vi "eyecat MAX v02_JS_140204.vi"() -> ()   [LabVIEW 2014]
doc: "This VI is an upgrade from the WIN 1_v4 that implements the ageing subrutine"
uses:
  <vilib>/Utility/file.llb/Write To Spreadsheet File (string).vi
  <vilib>/Utility/file.llb/Read From Spreadsheet File (string).vi
  <vilib>/regexp/Match Regular Expression.xnode
  Controls Win/Control 3.ctl
  <vilib>/Utility/miscctls.llb/LVRowAndColumnTypeDef.ctl
  <vilib>/Platform/TimedLoop/XDataNode/XDataNode.xnode
  <vilib>/Platform/TimedLoop/XDataNode/nitl_modes.ctl
  <vilib>/Platform/TimedLoop/XDataNode/XDNodeRunTimeDep.lvlib
  <vilib>/Platform/TimedLoop/XDataNode/wakeup.ctl
  <vilib>/Platform/TimedLoop/XDataNode/timing_clust.ctl
  Buttons/Numeric control.ctl
  <vilib>/Utility/file.llb/Read From Spreadsheet File (DBL).vi
  Buttons/String input.ctl
  Buttons/Numeric indicator.ctl
  Buttons/String output.ctl
panel:
  in  "MKS":bool
  out "output cluster":T2
  out "Lambda":dbl[](array[numeric])
  out "MKS HC":dbl
  in  "HC Index":i32
  in  "MFC Number":i32
  out "Open/Closed \nLoop":dbl[](array[numeric])
  out "Air Cyc 2":dbl[](array[numeric])
  in  "Cycle size":i32
  out "MFC Setpoint/Delivery":dynamicdata(graph)
  out "ExtAnDn":bool
  out "ExtAnUp":bool
  out "HC Cyc 2":dbl[](array[numeric])
  out "SO Valve 2":dbl[](array[numeric])
  out "SO Valve 1":dbl[](array[numeric])
  out "Air Bal":dbl[](array[numeric])
  out "HC Bal":dbl[](array[numeric])
  out "Air Cyc 1":dbl[](array[numeric])
  out "HC Cyc 1":dbl[](array[numeric])
  out "File name":string
  out "Log?":bool
  out "Advanced Logging":bool
  out "Connected":bool
  out "MKS 1":i16
  out "MKS 2":i16
  out "Furnace temp 2":dbl
  out "Full system?":bool
  out "Log interval (seconds)":T1
  in  "Flow rate Age":dbl
  in  "Inlet temp Age":dbl
  out "Stopped?":bool
  in  "Stop Cmd":T1
  out "Connected?":bool
  out "Error":dbl
  out "Iteration Duration":i64
  out "Finished Late? [i-1]":bool
  in  "stop TCP":bool
  in  "SO2 ppm":dbl
  out "Furnace temp 1":dbl
  out "stop 2":bool
  in  "Enum 1":i16=1
  in  "Acknowledge":bool
  out "Test number":u16
  out "Flag1":bool=TRUE
  out "EditPos Subc":T3
  out "Flag 2":bool=TRUE
  in  "Tab Control":T4(tab)
  out "Doors Unlocked":bool
  in  "Temperature Limit (°C)":T1=800.0 min=0.0 max=1200.0 step=1.0
  in  "Log Test Button":bool
  in  "File Name":T5="Test"
  in  "File Path":path=path "C:/DATA LOG"
  out "Fail":bool
  out "Pass":bool
  in  "Select Test Type":T6(radio)
  out "Standby":bool
  out "Doors Open":bool
  out "Extractor Fan On":bool
  out "Test In Progress":bool
  out "Cool Down":bool
  out "System Alarm":bool
  in  "Execute Leak Test Button":bool
  in  "Stop Test Button":bool
  in  "Start Test Button":bool
  in  "Advanced settings":bool
  in  "Inlet Temperature (°C)":T1=400.0 min=350.0 max=1000.0 step=1.0
  in  "Inlet LAMBDA Rich":T1=0.9 min=0.85 max=0.96 step=0.001
  in  "Inlet LAMBDA Lean":T1=1.2 min=1.02 max=3.0 step=0.001
  in  "Test Stop temperature (°C)":T1=300.0 min=100.0 max=1000.0 step=1.0
  in  "Test Start Temperature (°C)":T1=125.0 min=0.0 max=500.0 step=1.0
  in  "Furnace Ramp Rate (°C/min)":T1=15.0 min=1.0 max=50.0 step=0.1
  in  "NO:CO Ratio":T1=1.1 min=1.0 max=5.0 step=0.1
  in  "Inlet O2 (%)":T1=0.5 min=0.0 max=14.0 step=0.01
  in  "Inlet LAMBDA":T1=1.0 min=0.6 max=3.0 step=0.001
  out "Space Velocity (h-1)":T7
  out "Vol Flow @ STP (l/min)":T7
  in  "Test Flow Rate(g/s)":T1 min=0.0 max=100.0 step=0.01
  out "Sample Volume (litres)":T7
  in  "Number of Samples":T1=1.0 min=1.0 max=6.0 step=1.0
  in  "Sample Diameter (mm)":T1
  out "CO Theory (%)":T7 format="%#_3g"
  out "CO Theory (%)":T7 format="%#_3g"
  out "HC Theory (%)":T7
  in  "Sample Length (mm)":T1 min=0.0 step=0.5
  in  "NO ppm SW":dbl=500.0 caption="NO (ppm)" min=0.0 max=500.0 step=1.0
  in  "NO ppm Loff":T1 caption="NO ppm"
  in  "Delete sCycle":bool
  in  "Load sCycle":bool
  in  "Save sCycle":bool
  in  "Clear subcycle":bool
  in  "Clear Cycle Pattern":bool
  in  "Save Cycle":bool
  in  "Load Cycle":bool
  in  "Delete Cycle":bool
  out "Test Compiled":bool
  in  "Compile Test Button":bool
  in  "Sub-Cycle List":i32(listbox)=1
  in  "Cycle List":i32(listbox)=2
  out "Total Test Duration (hrs)":T8
  in  "Ageing Gas":enum32{"Radio Selection 1", "Radio Selection 2"}(radio)
  in  "Sub-Cycle Pattern":string[][](table) caption="Subcycle pattern"
  in  "Total Number of Cycles":T1=1.0 min=1.0 max=10000.0 step=1.0
  in  "Cycle Pattern":string[][](table)
  in  "Sub-Cycle Name":T5
  in  "Cycle Name":T5
  out "Heat Exchanger Temperatures (°C)":dynamicdata(graph)
  out "Flow Rate (g/s)":dynamicdata(graph)
  out "Sample Temperatures (°C)":dynamicdata(graph)
  out "System Temperatures (°C)":dynamicdata(graph)
  out "HC Concentration (ppm)":dynamicdata(graph)
  out "Lambda":dynamicdata(graph)
  out "M584L Upstream & Downstream":dynamicdata(graph)
  out "NO Concentration (ppm)":dynamicdata(graph)
  in  "Purge System":bool
  in  "Alarm ack":bool
  in  "Clear log":bool
  out "Table":string[][](table)
  out "Soft Alarm":bool
  out "Hard Alarm":bool
  # "0 HC Cyc 1\n1 Air Cyc 1\n2 Air Bal\n3 HC Bal\n4 Air Cyc 2\n5 HC Cyc 2"
  # "Test Type"
  # "Test Commands"
  # "System Indicators"
  # "Leak Test"
  # "Catalyst Specification"
  # "Lightoff Settings"
  # "Furnace Lightoff Settings"
  # "Sweep Settings"
  # "CO/HC Lightoff Settings"
  # "0.96 < lambda < 0.85"
  # "1.02< lambda < 1.6"
  # "350 < Tinlet < 1000"
  # "NO Lightoff Settings"
  # "Flow Specification"
  # "Cycle Compiled"
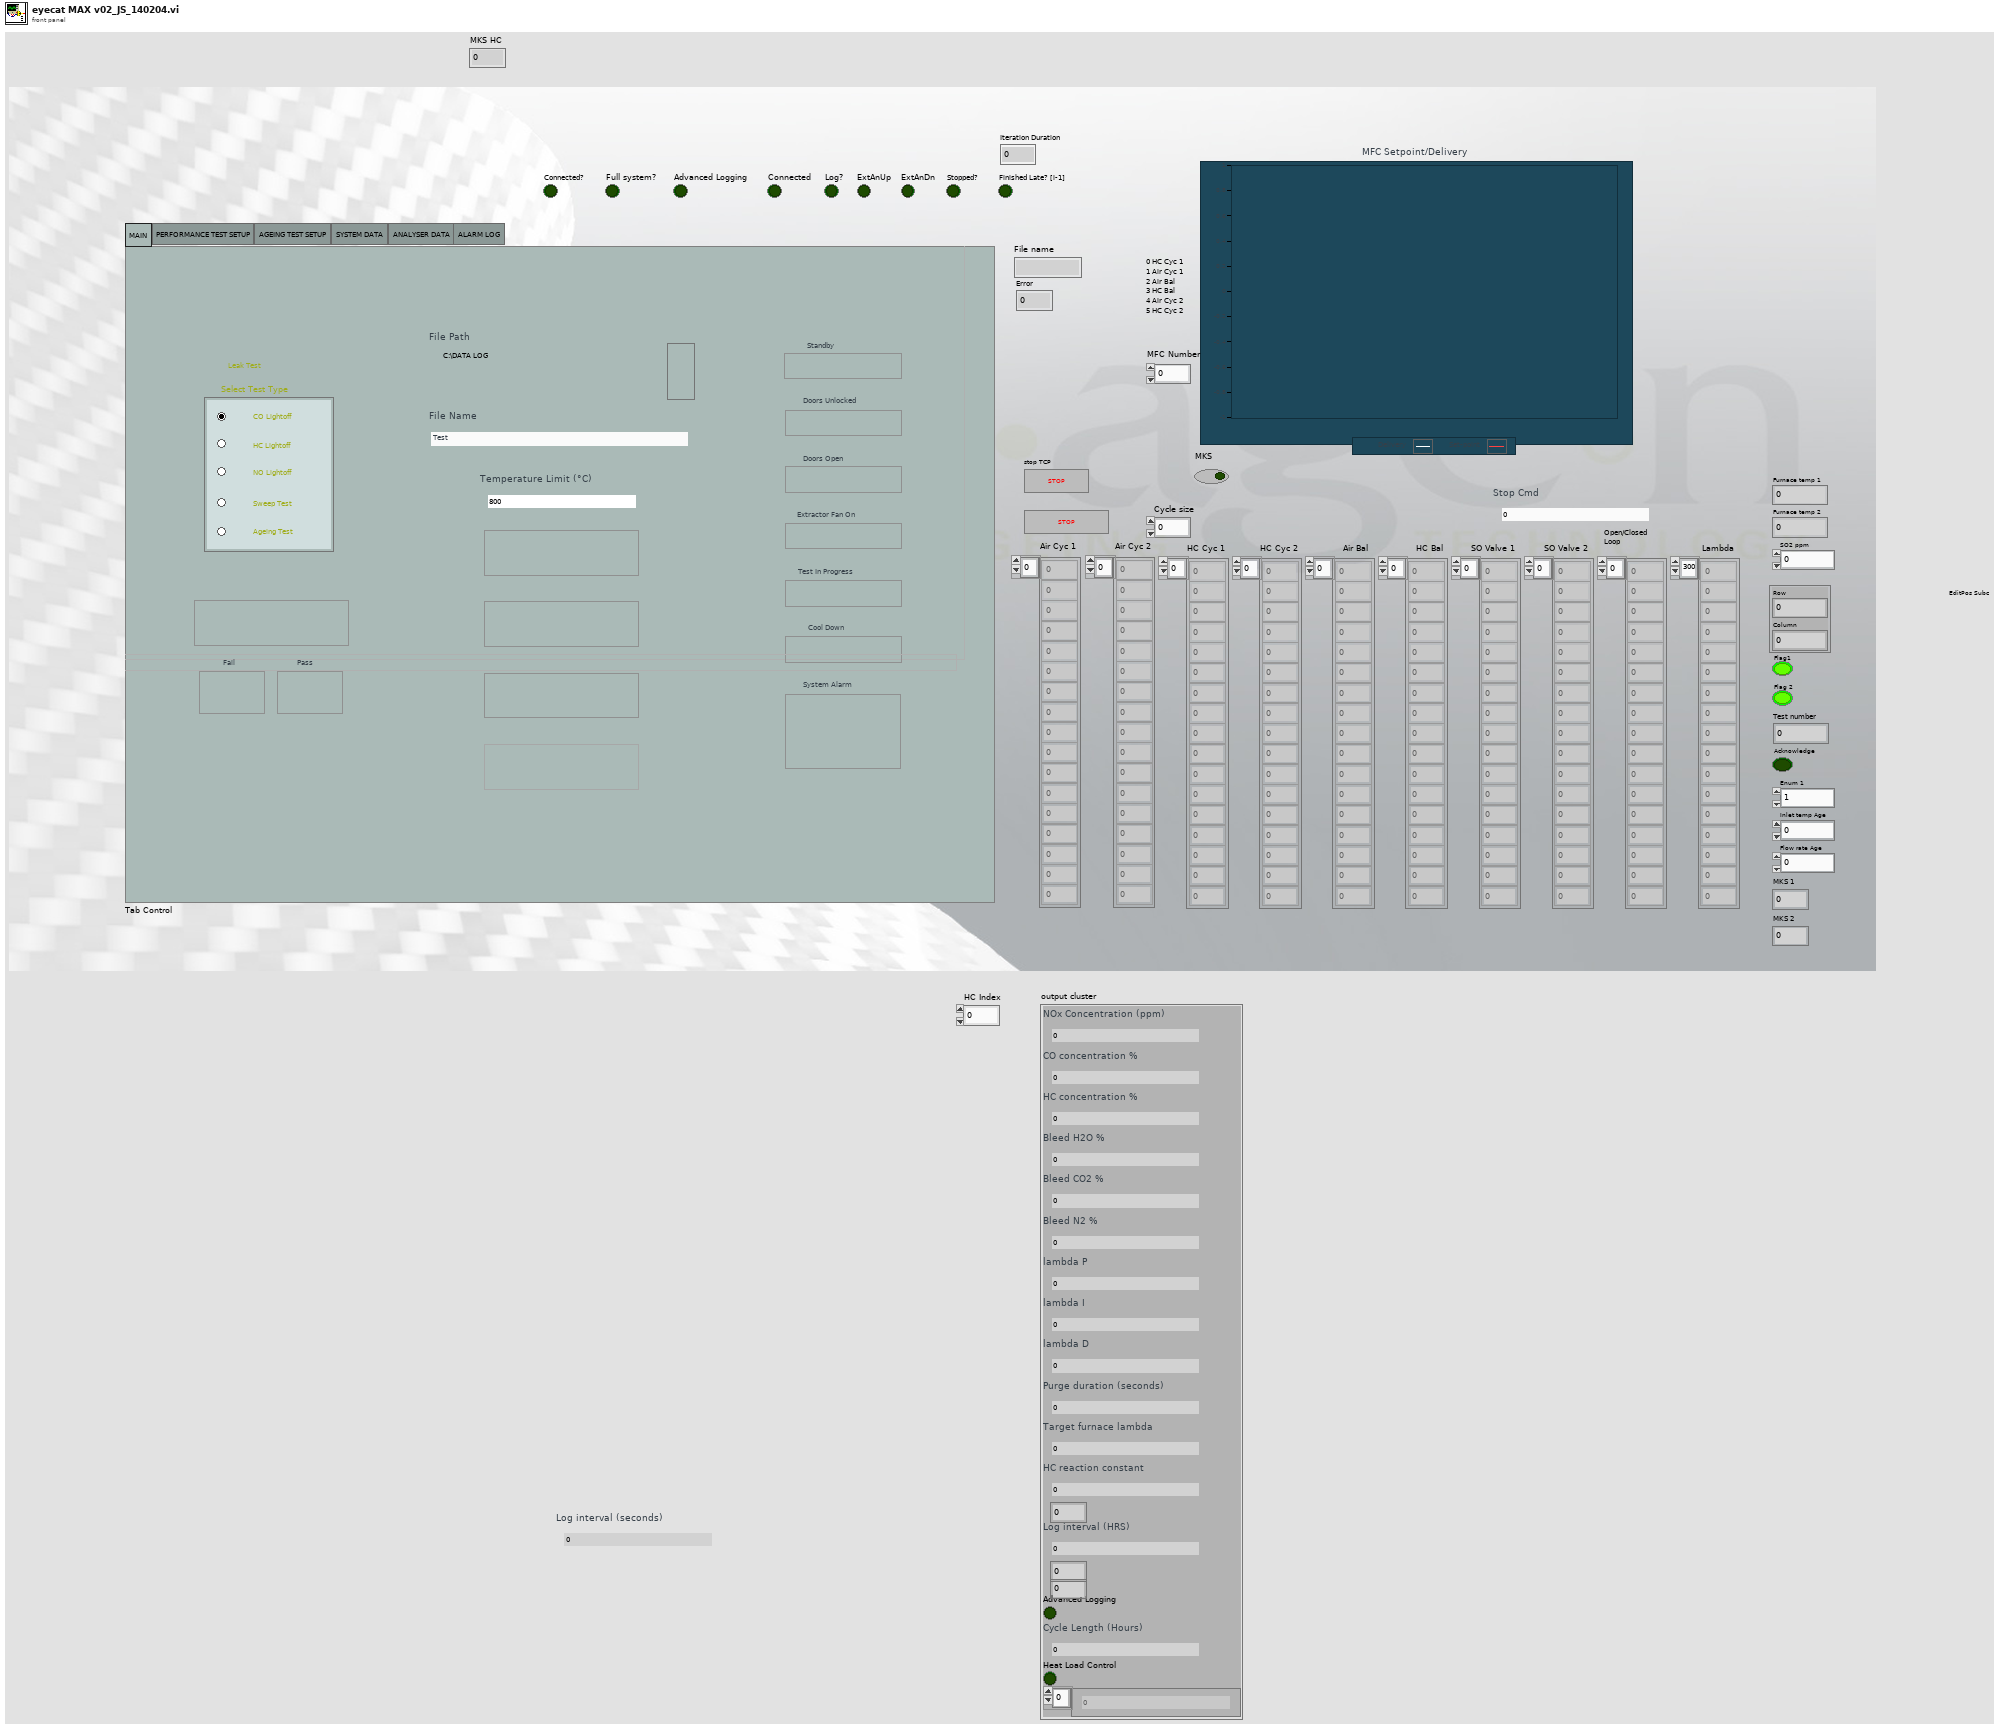
[diagram p1: front panel]
types:
  T1 = typedef "Numeric control.ctl" = dbl
  T2 = cluster{"NOx Concentration (ppm)":T1, "CO concentration %":T1, "HC concentration %":T1, "Bleed H2O %":T1, "Bleed CO2 %":T1, "Bleed N2 %":T1, "lambda P":T1, "lambda I":T1, "lambda D":T1, "Purge duration (seconds)":T1, "Target furnace lambda":T1, "HC reaction constant":T1, i16, "Log interval (HRS)":T1, i16, i16, "Advanced Logging":bool, "Cycle Length (Hours)":T1, "Heat Load Control":bool, T1[]}
  T3 = typedef "LVRowAndColumnTypeDef.ctl" = cluster{"Row":i32, "Column":i32}
  T4 = enum32{"MAIN", "PERFORMANCE TEST SETUP", "AGEING TEST SETUP", "SYSTEM DATA", "ANALYSER DATA", "ALARM LOG"}
  T5 = typedef "String input.ctl" = string
  T6 = enum32{"CO Lightoff", "HC Lightoff", "NO Lightoff", "Sweep Test", "Ageing Test"}
  T7 = typedef "Numeric indicator.ctl" = dbl
  T8 = typedef "String output.ctl" = string
  T9 = typedef "XDNodeRunTimeDep.lvlib/nitl_modes.ctl" = enum32{"No Change", "Process missed periods, maintain original phase", "Discard missed periods, maintain original phase", "Process missed periods, ignore original phase", "Discard missed periods, ignore original phase"}
  T10 = typedef "Control 3.ctl" = enum16{"main", "start test", "save subc", "load subc", "delete subc", "clear table 1", "update list 1", "save cycle", "load cycle", "delete cycle", "clear table 2", "update list 2", "calc HC CO", "Total time calc", "update Cycle pattern ", "load cycle name", "convert to num", "load test array", "check scycle name", "check cycle name", "Multigas connect", "Multigas disconnect"}
  T11 = enum8{"Enabled", "Disabled", "Disabled and Grayed Out"}
  T12 = typedef "XDNodeRunTimeDep.lvlib/timing_clust.ctl" = cluster{"Expected End [f-1]":u64, "Actual End [f-1]":u64, "Finished Late? [f-1]":bool, "Expected End [i-1]":u64, "Actual End [i-1]":u64, "Finished Late? [i-1]":bool, "Expected Start [i]":u64, "Actual Start [i]":u64, "Expected Start [f]":u64, "Actual Start [f]":u64, "Source Name":string, "Structure Name":string, "Period":i64, "Deadline":i64, "Offset":i64, "Start":i64, "Priority":i32, "Timeout":i32, "Mode":T9, "Wakeup Reason":T13, "Error":errorcluster, "Source Type":string, "Secondary Source Type":string, "Global End Time":u64, "Global Start Time":u64, "Frame Duration":u64, "Iteration Duration":u64, "Assigned CPU":i32, "I/O Scan Engine Mode":u32}
  T13 = typedef "XDNodeRunTimeDep.lvlib/wakeup.ctl" = enum32{"Normal", "Aborted", "Asynchronous wakeup", "Timing source error", "Timed loop error", "Timeout"}
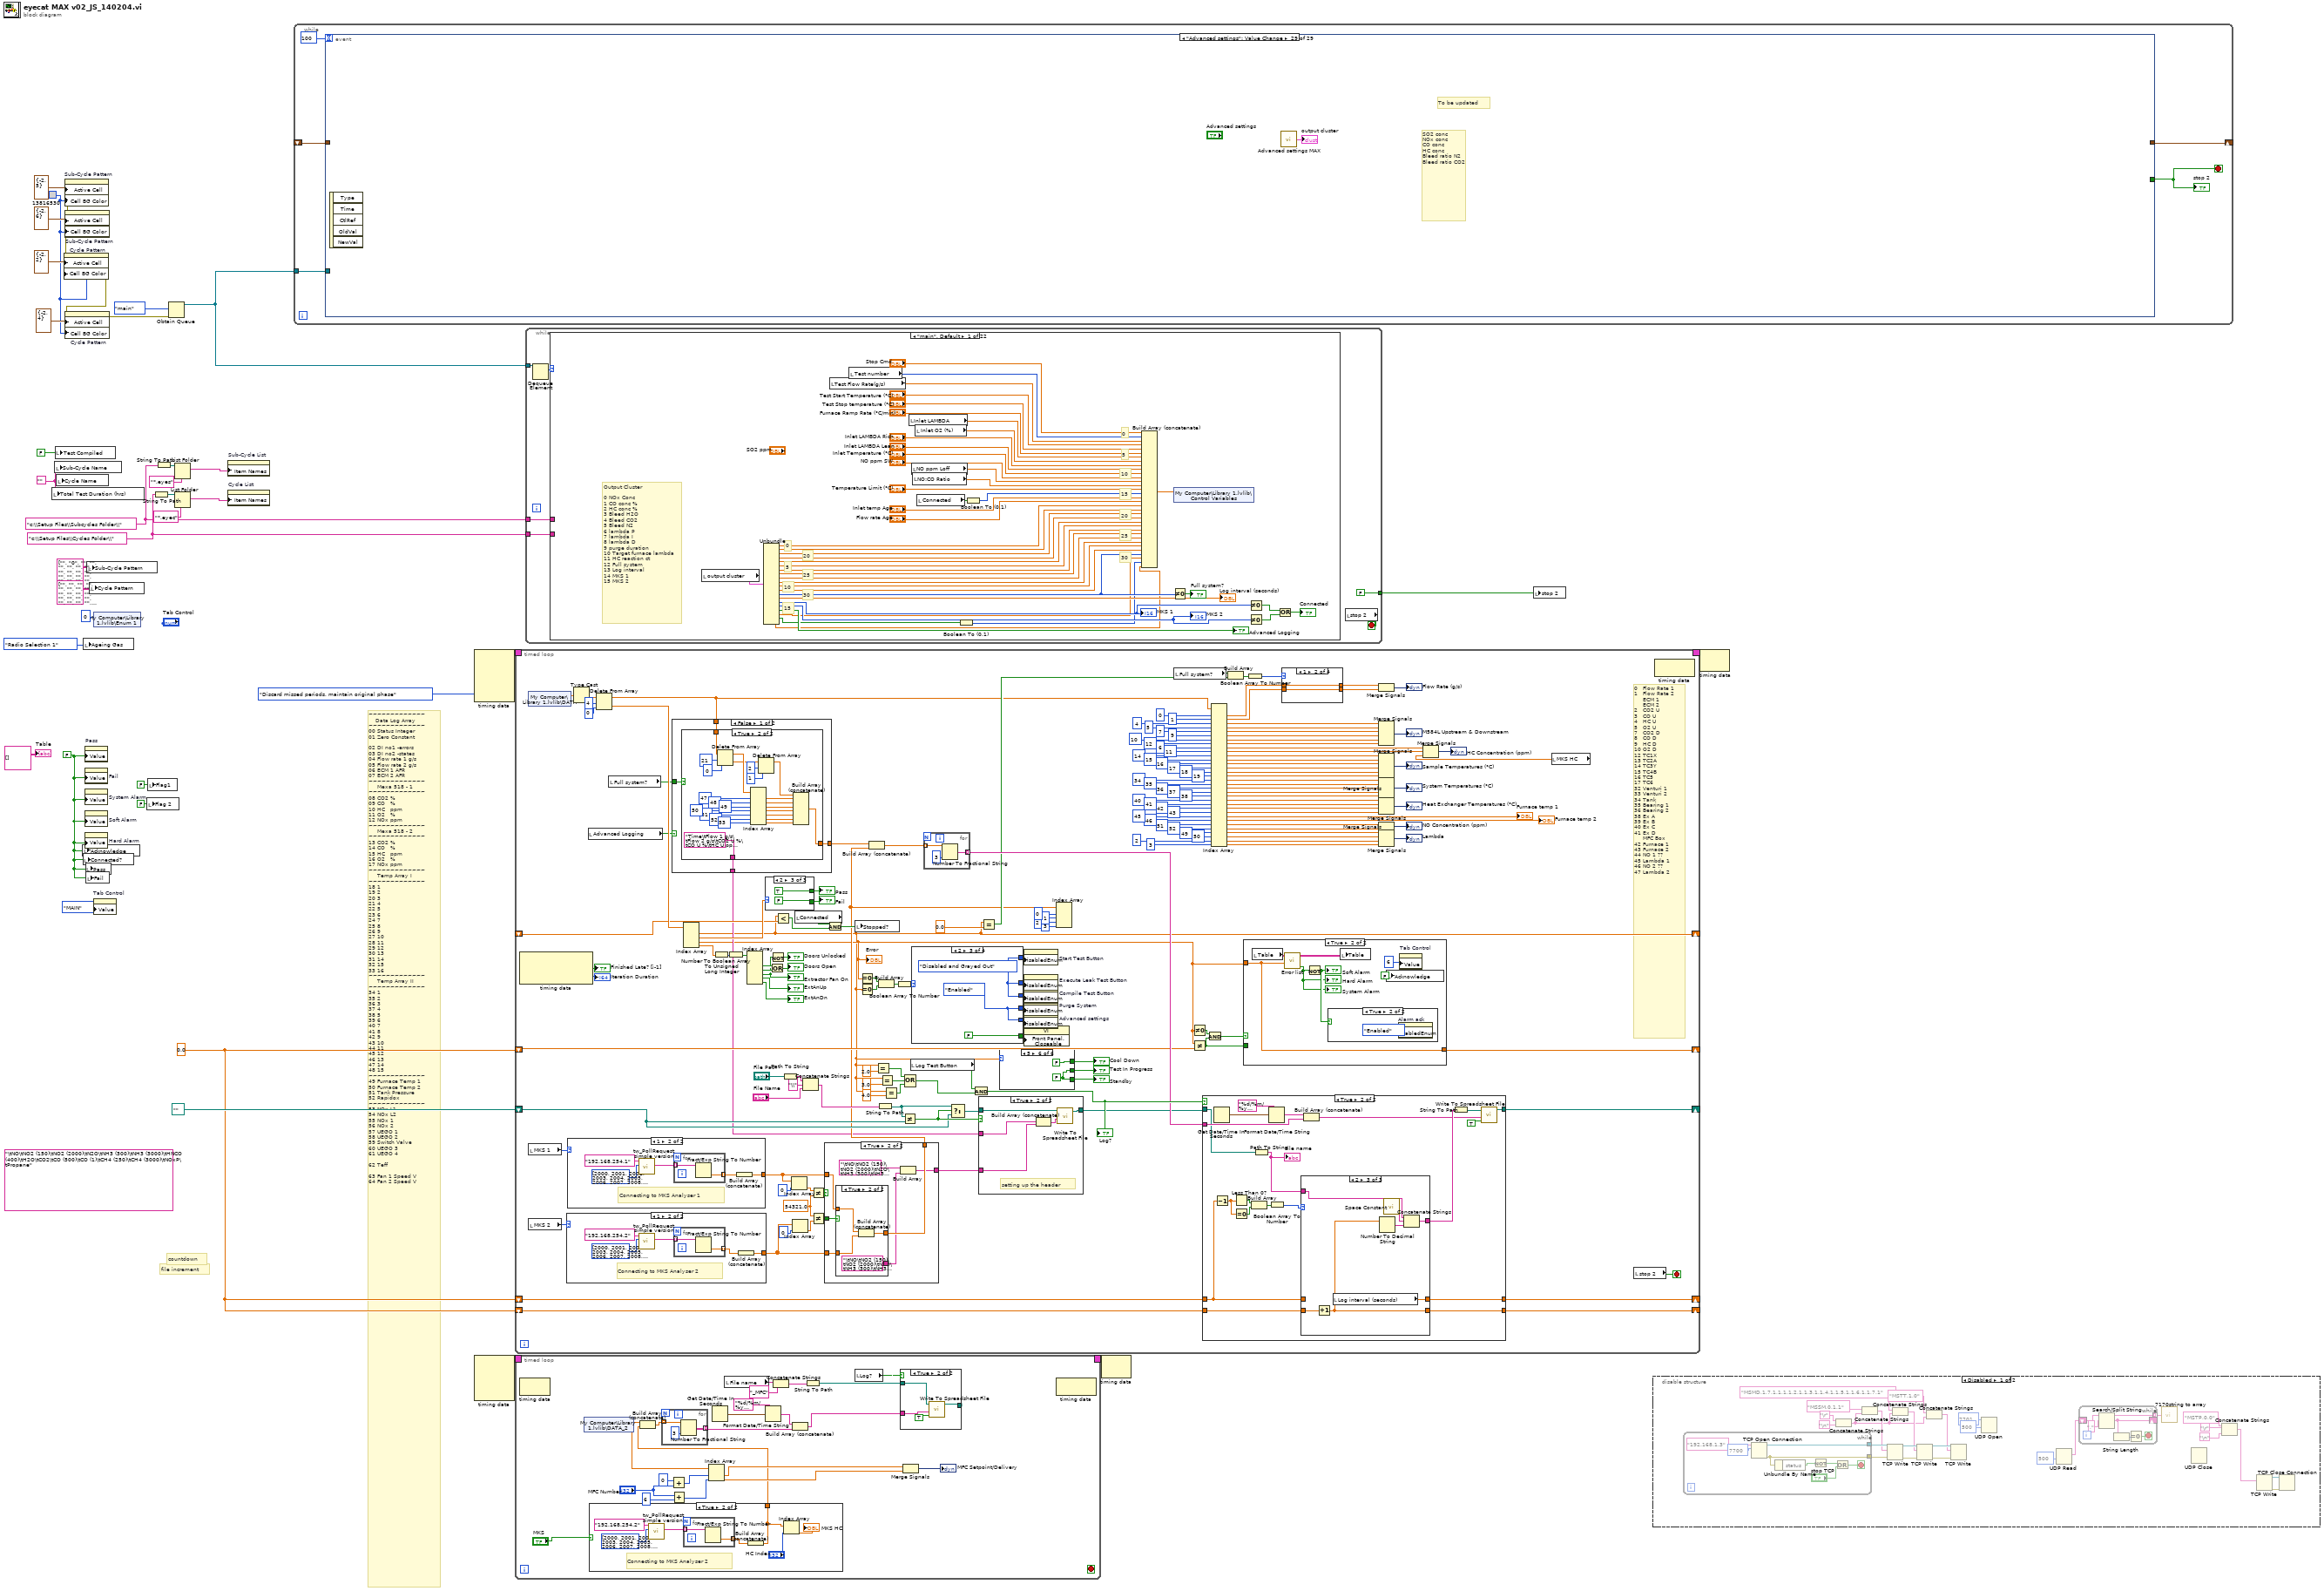
[diagram p0: block diagram]
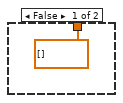
[diagram p2: hidden frame]
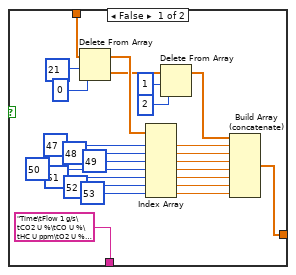
[diagram p5: hidden frame]
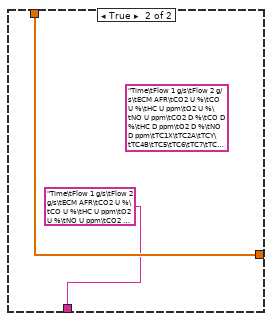
[diagram p6: hidden frame]
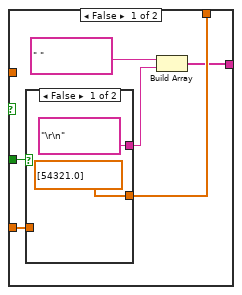
[diagram p7: hidden frame]
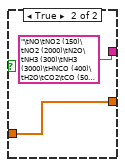
[diagram p8: hidden frame]
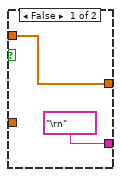
[diagram p9: hidden frame]
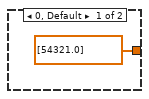
[diagram p10: hidden frame]
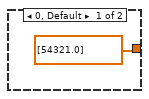
[diagram p11: hidden frame]
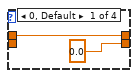
[diagram p12: hidden frame]
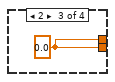
[diagram p13: hidden frame]
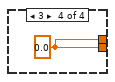
[diagram p14: hidden frame]
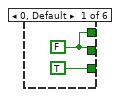
[diagram p15: hidden frame]
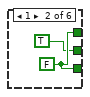
[diagram p16: hidden frame]
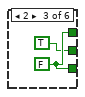
[diagram p17: hidden frame]
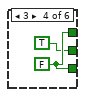
[diagram p18: hidden frame]
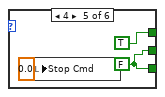
[diagram p19: hidden frame]
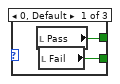
[diagram p20: hidden frame]
diagram:
  (unwired) "\tNO\tNO2 (150)\tNO2 (2000)\tN2O\tNH3 (300)\tNH3 (3000)\tHNCO (400)\tH2O\tCO2\tCO (500)\tCO (1)\tCH4 (250)\tCH4 (3000)\tNOxP\tPropane" ("Heading string 2")
  w4 = FALSE
  w3 = 0.0 ("y")
  w20 = ""
  w23 = "c:\\Setup Files\\Cycles Folder\\"
  w29 = u32 13816530
  w21 = "c:\\Setup Files\\Subcycles Folder\\"
  # "~~~~~~~~~~~~~\n    Data Log Array\n~~~~~~~~~~~~~\n00 Status Integer\n01 Zero Constant\n\n02 DI no1 -errors\n03 DI no2 -states\n04 Flow rate 1 g/s\n05 Flow rate 2 g/s\n06 ECM 1 AFR\n07 ECM 2 AFR\n~~~~~~~~~~~~~\n     Mexa 518 - 1\n~~~~~~~~~~~~~\n08 CO2 %\n09 CO   %\n10 HC   ppm\n11 O2   %\n12 NOx ppm\n~~~~~~~~~~~~~\n     Mexa 518 - 2\n~~~~~~~~~~~~~\n13 CO2 %\n14 CO   %\n15 HC   ppm\n16 O2   %\n17 NOx ppm\n~~~~~~~~~~~~~\n     Temp Array I\n~~~~~~~~~~~~~\n18 1\n19 2 \n20 3\n21 4\n22 5\n23 6\n24 7\n25 8\n26 9\n27 10\n28 11\n29 12\n30 13\n31 14\n32 15\n33 16\n~~~~~~~~~~~~~\n     Temp Array II\n~~~~~~~~~~~~~\n34 1\n35 2\n36 3\n37 4\n38 5\n39 6\n40 7\n41 8\n42 9\n43 10\n44 11\n45 12\n46 13\n47 14\n48 15\n~~~~~~~~~~~~~\n49 Furnace Temp 1\n50 Furnace Temp 2\n51 Tank Pressure\n52 Rapidox\n~~~~~~~~~~~~~\n53 NOx L1\n54 NOx L2\n55 NOx 1\n56 NOx 2\n57 UEGO 1\n58 UEGO 2\n59 Switch Valve\n60 UEGO 3\n61 UEGO 4\n\n62 Teff\n\n63 Fan 1 Speed V\n64 Fan 2 Speed V"
  # "file increment"
  # "countdown"
  n1 = local write "Total Test Duration (hrs)"(w20) -> ()
  n2 = local write "Sub-Cycle Name"(w20) -> ()
  n3 = local write "Test Compiled"(FALSE ("Cycle Compiled")) -> ()
  n4 = local write "Cycle Name"(w20) -> ()
  n5 = property on="Sub-Cycle Pattern" class="Tbl (strict)"("Active Cell"=T3 {"Row"=-2, "Column"=5} ("Active Cell:Active Cell"), "Cell BG Color"=w29) -> (error out=w34:errorcluster)  [unwired: 2 in, 1 out]
  n6 = property on="Sub-Cycle Pattern" class="Tbl (strict)"(error in=w34, "Active Cell"=T3 {"Row"=-2, "Column"=6} ("Active Cell:Active Cell"), "Cell BG Color"=w29) -> (error out=w33:errorcluster)  [unwired: 1 in, 1 out]
  n7 = property on="Cycle Pattern" class="Tbl (strict)"(error in=w33, "Active Cell"=T3 {"Row"=-2, "Column"=2} ("Active Cell:Active Cell"), "Cell BG Color"=w29) -> (error out=w31:errorcluster)  [unwired: 1 in, 1 out]
  n8 = property on="Cycle Pattern" class="Tbl (strict)"(error in=w31, "Active Cell"=T3 {"Row"=-2, "Column"=4} ("Active Cell:Active Cell"), "Cell BG Color"=w29) -> (error out=w28:errorcluster)  [unwired: 1 in, 1 out]
  n9 = local write "Acknowledge"(w4) -> ()
  n10 = local write "Connected?"(w4) -> ()
  n11 = local write "Ageing Gas"(enum32{"Radio Selection 1", "Radio Selection 2"}."Radio Selection 1" ("Ageing Gas")) -> ()
  n12 = property on="Pass" class="Bool (strict)"("Value"=w4) -> ()  [unwired: 2 in, 2 out]
  n13 = property on="Fail" class="Bool (strict)"("Value"=w4) -> ()  [unwired: 2 in, 2 out]
  n14 = property on="System Alarm" class="Bool (strict)"("Value"=w4) -> ()  [unwired: 2 in, 2 out]
  n15 = property on="Soft Alarm" class="Bool (strict)"("Value"=w4) -> ()  [unwired: 2 in, 2 out]
  n16 = property on="Hard Alarm" class="Bool (strict)"("Value"=w4) -> ()  [unwired: 2 in, 2 out]
  n17 = local write "Pass"(w4) -> ()
  n18 = local write "Fail"(w4) -> ()
  n19 = local write "Sub-Cycle Pattern"(string[][] [["", "0", "", "", "", "", "", "", "", "", "", "", ""], ["", "", "", "", "", "", "", "", "", "", "", "", ""], ["", "", "", "", "", "", "", "", "", "", "", "", ""], ["", "", "", "", "", "", "", "", "", "", "", "", ""], ["", "", "", "", "", "", "", "", "", "", "", "", ""], ["", "", "", "", "", "", "", "", "", "", "", "", ""], ["", "", "", "", "", "", "", "", "", "", "", "", ""], ["", "", "", "", "", "", "", "", "", "", "", "", ""], ["", "", "", "", "", "", "", "", "", "", "", "", ""], ["", "", "", "", "", "", "", "", "", "", "", "", ""], ["", "", "", "", "", "", "", "", "", "", "", "", ""], ["", "", "", "", "", "", "", "", "", "", "", "", ""], ["", "", "", "", "", "", "", "", "", "", "", "", ""], ["", "", "", "", "", "", "", "", "", "", "", "", ""], ["", "", "", "", "", "", "", "", "", "", "", "", ""], ["", "", "", "", "", "", "", "", "", "", "", "", ""], ["", "", "", "", "", "", "", "", "", "", "", "", ""], ["", "", "", "", "", "", "", "", "", "", "", "", ""], ["", "", "", "", "", "", "", "", "", "", "", "", ""], ["", "", "", "", "", "", "", "", "", "", "", "", ""], ["", "", "", "", "", "", "", "", "", "", "", "", ""], ["", "", "", "", "", "", "", "", "", "", "", "", ""], ["", "", "", "", "", "", "", "", "", "", "", "", ""], ["", "", "", "", "", "", "", "", "", "", "", "", ""], ["", "", "", "", "", "", "", "", "", "", "", "", ""], ["", "", "", "", "", "", "", "", "", "", "", "", ""], ["", "", "", "", "", "", "", "", "", "", "", "", ""], ["", "", "", "", "", "", "", "", "", "", "", "", ""], ["", "", "", "", "", "", "", "", "", "", "", "", ""], ["", "", "", "", "", "", "", "", "", "", "", "", ""], ["", "", "", "", "", "", "", "", "", "", "", "", ""]]) -> ()
  n20 = local write "Cycle Pattern"(string[][] [["", "", "", "", ""], ["", "", "", "", ""], ["", "", "", "", ""], ["", "", "", "", ""], ["", "", "", "", ""], ["", "", "", "", ""], ["", "", "", "", ""], ["", "", "", "", ""], ["", "", "", "", ""], ["", "", "", "", ""], ["", "", "", "", ""], ["", "", "", "", ""], ["", "", "", "", ""], ["", "", "", "", ""], ["", "", "", "", ""], ["", "", "", "", ""], ["", "", "", "", ""], ["", "", "", "", ""], ["", "", "", "", ""], ["", "", "", "", ""], ["", "", "", "", ""], ["", "", "", "", ""], ["", "", "", "", ""], ["", "", "", "", ""], ["", "", "", "", ""], ["", "", "", "", ""], ["", "", "", "", ""], ["", "", "", "", ""], ["", "", "", "", ""], ["", "", "", "", ""], ["", "", "", "", ""]]) -> ()
  n21 = shared-variable "My Computer\\Library 1.lvlib\\Enum 1"(u16 0 ("Enum 1")) -> ()  [unwired: 1 in, 1 out]
  n22 = property on="Tab Control" class="TabCtl (strict)"("Value"=T4."MAIN" ("Tab Control")) -> ()  [unwired: 2 in, 2 out]
  n23 = local write "Flag 2"(FALSE) -> ()
  n24 = local write "Flag1"(FALSE) -> ()
  n25 = String To Path(string=w23) -> (path=w24:path)
  n26 = String To Path(string=w21) -> (path=w26:path)
  n27 = Obtain Queue(element data type=Control_3."main" ("Enum"), error in (no error)=w28) -> (queue out=w37:refnum<queue>)  [unwired: 3 in, 2 out]
  n28 = List Folder(path=w24, pattern="*.eyec") -> (filenames=w25:string[])  [unwired: 2 in, 3 out]
  n29 = List Folder(path=w26, pattern="*.eyes") -> (filenames=w27:string[])  [unwired: 2 in, 3 out]
  n30 = property on="Sub-Cycle List" class="LstBox (strict)"("Item Names"=w27) -> ()  [unwired: 2 in, 2 out]
  n31 = property on="Cycle List" class="LstBox (strict)"("Item Names"=w25) -> ()  [unwired: 2 in, 2 out]
  n32 = while {
    tunnel: w37 -> [w43]
    shift-right: [w41] -> _
    shift-left: _ -> [w40]
    stop <- w39 stop-if-true
    n33 = event shown="[28] \"Advanced settings\": Value Change" {
      selector: _ -> [_ _ _ _ _ _ _ _ _ _ _ _ _ _ _ _ _ _ _ _ _ _ _ _ _ _ _ _ _]
      dyn-events: _ -> [_ _ _ _ _ _ _ _ _ _ _ _ _ _ _ _ _ _ _ _ _ _ _ _ _ _ _ _ _]
      timeout: 100 -> [_ _ _ _ _ _ _ _ _ _ _ _ _ _ _ _ _ _ _ _ _ _ _ _ _ _ _ _ _]
      tunnel: w43 -> [w46 w48 _ w57 w65 w72 w79 w90 w94 w105 w110 w113 w118 w140 w148 w149 _ _ _ _ w193 w209 _ w286 w304 _ w318 _ _]
      tunnel: [w44 w47 _ w58 w64 w71 w78 w89 w92 w100 w107 w112 w116 w137 _ _ _ _ _ _ _ _ _ _ _ _ _ _ _] -> w41
      tunnel: w40 -> [w44 w47 _ w58 w64 w71 w77 w89 w92 w100 w107 w112 w116 w137 _ _ _ _ _ _ _ _ _ _ _ _ _ _ _]
      tunnel: [_ _ w50 _ _ _ _ _ _ _ _ _ _ _ _ _ _ _ _ _ _ _ _ _ _ _ _ _ _] -> w39
      event Timeout {
        n34 = event-data() -> ()  [unwired: 1 in, 2 out]
        n35 = Enqueue Element(queue=w46, element=Control_3."main" ("Enum")) -> ()  [unwired: 2 in, 3 out]
      }
      event "Clear subcycle": Value Change {
        n36 = event-data() -> ()  [unwired: 1 in, 5 out]
        n37 = Enqueue Element(queue=w48, element=Control_3."clear table 1" ("Enum")) -> ()  [unwired: 2 in, 3 out]
      }
      event Panel Close? {
        n38 = event-data() -> ()  [unwired: 1 in, 3 out]
        n39 = Two Button Dialog(message="This command will close Eyecat!\nDo you wish to continue?", 1:"No" ("F button name (\"Cancel\")"), 2:"Yes" ("T button name (\"OK\")")) -> (T button?=w50:bool)
        n40 = Not(x=w50) -> (.not. x?=w51:bool)
        n41 = event-data("Discard?"=w51) -> ()  [unwired: 1 in, 1 out]
      }
      event "Save sCycle": Value Change {
        n42 = event-data() -> ()  [unwired: 1 in, 5 out]
        n43 = local read "Sub-Cycle Pattern"() -> (w55:string[][])
        n44 = call "Time column check.vi"("Array"=w55) -> ("Mistake?"=w56:bool)  [unwired: 10 in]
        n45 = case shown="False" w56 {
          tunnel: w57 -> [w59 _]
          frame False {
            n46 = Enqueue Element(queue=w59, element=Control_3."save subc") -> (queue out=w61:refnum<queue>)  [unwired: 2 in, 2 out]
            n47 = Enqueue Element(queue=w61, element=Control_3."update list 1") -> ()  [unwired: 2 in, 3 out]
          }
          frame True {
            n48 = One Button Dialog(message="The time sequence is incorrect!\nReview and save again!") -> ()  [unwired: 1 in, 1 out]
          }
        }
      }
      event "Load sCycle": Value Change {
        n49 = event-data() -> ()  [unwired: 1 in, 5 out]
        n50 = Enqueue Element(queue=w65, element=Control_3."load subc") -> ()  [unwired: 2 in, 3 out]
      }
      event "Delete sCycle": Value Change {
        n51 = event-data() -> ()  [unwired: 1 in, 5 out]
        n52 = Enqueue Element(queue=w72, element=Control_3."delete subc") -> (queue out=w74:refnum<queue>)  [unwired: 2 in, 2 out]
        n53 = Enqueue Element(queue=w74, element=Control_3."update list 1") -> (queue out=w70:refnum<queue>)  [unwired: 2 in, 2 out]
        n54 = Enqueue Element(queue=w70, element=Control_3."update Cycle pattern ") -> (queue out=w67:refnum<queue>)  [unwired: 2 in, 2 out]
        n55 = Enqueue Element(queue=w67, element=Control_3."Total time calc") -> ()  [unwired: 2 in, 3 out]
      }
      event "Sub-Cycle Pattern": Mouse Down; "Sub-Cycle Pattern": Value Change {
        n56 = event-data() -> ()  [unwired: 1 in, 3 out]
        n57 = property on="Sub-Cycle Pattern" class="Tbl (strict)"() -> ("EditPos"=w78:T3)  [unwired: 2 in, 2 out]
        n58 = Unbundle By Name(w78) -> ("Row"=w80:i32)  [unwired: 1 out]
        n59 = Less?(x=w80, y=30) -> (x < y?=w82:bool)
        n60 = case shown="True" w82 {
          tunnel: w79 -> [_ w87]
          frame False {
            n61 = One Button Dialog(message="This table is limited to 30 entries!") -> ()  [unwired: 1 in, 1 out]
          }
          frame True {
            n62 = Enqueue Element(queue=w87, element=Control_3."convert to num") -> (queue out=w86:refnum<queue>)  [unwired: 2 in, 2 out]
            n63 = Enqueue Element(queue=w86, element=Control_3."calc HC CO") -> ()  [unwired: 2 in, 3 out]
          }
        }
        "EditPos Subc" <- w77
        "Flag1" <- TRUE
      }
      event "Clear Cycle Pattern": Value Change {
        n64 = event-data() -> ()  [unwired: 1 in, 5 out]
        n65 = Enqueue Element(queue=w90, element=Control_3."clear table 2" ("Enum")) -> ()  [unwired: 2 in, 3 out]
        n66 = local write "Test Compiled"(FALSE ("Test Compiled")) -> ()
      }
      event "Save Cycle": Value Change {
        n67 = event-data() -> ()  [unwired: 1 in, 5 out]
        n68 = Enqueue Element(queue=w94, element=Control_3."update Cycle pattern ") -> (queue out=w93:refnum<queue>)  [unwired: 2 in, 2 out]
        n69 = Enqueue Element(queue=w93, element=Control_3."save cycle") -> (queue out=w97:refnum<queue>)  [unwired: 2 in, 2 out]
        n70 = Enqueue Element(queue=w97, element=Control_3."update list 2") -> ()  [unwired: 2 in, 3 out]
      }
      event "Load Cycle": Value Change {
        n71 = event-data() -> ()  [unwired: 1 in, 5 out]
        n72 = Enqueue Element(queue=w105, element=Control_3."load cycle") -> (queue out=w103:refnum<queue>)  [unwired: 2 in, 2 out]
        n73 = Enqueue Element(queue=w103, element=Control_3."update Cycle pattern ") -> (queue out=w102:refnum<queue>)  [unwired: 2 in, 2 out]
        n74 = local write "Test Compiled"(FALSE ("Test Compiled")) -> ()
        n75 = Enqueue Element(queue=w102, element=Control_3."Total time calc") -> ()  [unwired: 2 in, 3 out]
      }
      event "Delete Cycle": Value Change {
        n76 = event-data() -> ()  [unwired: 1 in, 5 out]
        n77 = Enqueue Element(queue=w110, element=Control_3."delete cycle") -> (queue out=w109:refnum<queue>)  [unwired: 2 in, 2 out]
        n78 = Enqueue Element(queue=w109, element=Control_3."update list 2") -> ()  [unwired: 2 in, 3 out]
      }
      event Value Change {
        n79 = event-data() -> ()  [unwired: 1 in, 5 out]
        n80 = Enqueue Element(queue=w113, element=Control_3."Total time calc") -> ()  [unwired: 2 in, 3 out]
      }
      event "Cycle Pattern": Mouse Up; "Cycle Pattern": Value Change {
        n81 = event-data() -> ()  [unwired: 1 in, 3 out]
        n82 = property on="Cycle Pattern" class="Tbl (strict)"() -> ("EditPos"=w120:T3)  [unwired: 2 in, 2 out]
        n83 = Unbundle By Name(w120) -> ("Row"=w117:i32, "Column"=w122:i32)
        n84 = Less?(x=w117, y=30) -> (x < y?=w121:bool)
        n85 = case shown="True" w121 {
          tunnel: w122 -> [_ w124]
          tunnel: w118 -> [_ w127]
          frame False {
            n86 = One Button Dialog(message="This table is limited to 30 entries!") -> ()  [unwired: 1 in, 1 out]
          }
          frame True {
            n87 = Equal?(x=w124, y=1) -> (x = y?=w128:bool)
            n88 = case shown="True" w128 {
              tunnel: w127 -> [w131 w134]
              tunnel: [w130 w133] -> w126
              frame False {
                n89 = Enqueue Element(queue=w131, element=Control_3."update Cycle pattern ") -> (queue out=w130:refnum<queue>)  [unwired: 2 in, 2 out]
              }
              frame True {
                n90 = Enqueue Element(queue=w134, element=Control_3."load cycle name") -> (queue out=w133:refnum<queue>)  [unwired: 2 in, 2 out]
              }
            }
            n91 = Enqueue Element(queue=w126, element=Control_3."Total time calc") -> ()  [unwired: 2 in, 3 out]
          }
        }
        "Flag 2" <- TRUE
      }
      event "Compile Test Button": Value Change {
        n92 = event-data() -> ()  [unwired: 1 in, 5 out]
        n93 = local read "Flag 2"() -> (w136:bool)
        n94 = case shown="True" w136 {
          tunnel: w140 -> [w141 w145]
          tunnel: [w141 w142] -> w138
          frame False {
          }
          frame True {
            n95 = Enqueue Element(queue=w145, element=Control_3."save cycle") -> (queue out=w143:refnum<queue>)  [unwired: 2 in, 2 out]
            n96 = Enqueue Element(queue=w143, element=Control_3."update list 2") -> (queue out=w142:refnum<queue>)  [unwired: 2 in, 2 out]
          }
        }
        n97 = Enqueue Element(queue=w138, element=Control_3."load test array") -> ()  [unwired: 2 in, 3 out]
      }
      event Value Change {
        n98 = event-data() -> ()  [unwired: 1 in, 5 out]
        n99 = Enqueue Element(queue=w148, element=Control_3."check scycle name") -> ()  [unwired: 2 in, 3 out]
      }
      event Value Change {
        n100 = event-data() -> ()  [unwired: 1 in, 5 out]
        n101 = Enqueue Element(queue=w149, element=Control_3."check cycle name") -> ()  [unwired: 2 in, 3 out]
      }
      event Value Change {
        n102 = event-data() -> ()  [unwired: 1 in, 5 out]
        n103 = Square(x="Sample Diameter (mm)") -> (x^2=w158:T1)
        n104 = Compound Arithmetic op=MULTIPLY(w158, "Sample Length (mm)", "Number of Samples", 3.141592653589793) -> (w157:T1)
        n105 = Divide(x=w157, y=4000000.0) -> (x/y=→"Sample Volume (litres)":T1)
      }
      event Value Change {
        # "O2Eq"
        n106 = event-data() -> ()  [unwired: 1 in, 5 out]
        n107 = local write "Inlet LAMBDA"("Inlet LAMBDA") -> ()
        n108 = local write "Inlet O2 (%)"("Inlet O2 (%)") -> ()
        n109 = Decrement(x="Inlet LAMBDA") -> (x-1=w173:T1)
        n110 = Multiply(x=4.76, y="Inlet LAMBDA") -> (x*y=w169:T1)
        n111 = Multiply(x=w173, y=100.0) -> (x*y=w171:T1)
        n112 = Add(x=0.33, y=w169) -> (x+y=w167:T1)
        n113 = Divide(x=w171, y=w167) -> (x/y=w166:T1)
        n114 = Subtract(x="Inlet O2 (%)", y=w166) -> (x-y=w164:T1)
        n115 = Multiply(x=w164, y=2.0) -> (x*y=→"CO Theory (%)":T1)
        n116 = Divide(x=w164, y=4.5) -> (x/y=→"HC Theory (%)":T1)
      }
      event Value Change {
        n117 = event-data() -> ()  [unwired: 1 in, 5 out]
        n118 = local write "NO ppm Loff"("NO ppm Loff") -> ()
        n119 = local write "NO:CO Ratio"("NO:CO Ratio") -> ()
        n120 = Divide(x="NO ppm Loff", y=T1 10000.0) -> (x/y=w176:T1)
        n121 = Multiply(x="NO:CO Ratio", y=w176) -> (x*y=→"CO Theory (%)":T1)
      }
      event Value Change {
        n122 = event-data() -> ()  [unwired: 1 in, 5 out]
        n123 = local read "Sample Volume (litres)"() -> (w181:T7)
        n124 = Equal?(x=w181, y=0.0) -> (x = y?=w180:bool)
        n125 = case shown="False" w180 {
          tunnel: w181 -> [w186 _]
          tunnel: "Test Flow Rate(g/s)" -> [w183 _]
          frame False {
            w188 = 60.0 ("y")
            n126 = Multiply(x=w183, y=w188) -> (x*y=w190:T1)
            n127 = Divide(x=w190, y=1.2) -> (x/y=w185:T1)
            "Vol Flow @ STP (l/min)" <- w185
            n128 = Multiply(x=w185, y=w188) -> (x*y=w187:T1)
            n129 = Divide(x=w187, y=w186) -> (x/y=→"Space Velocity (h-1)":T1)
          }
          frame True {
            n130 = One Button Dialog(message="Review sample specification first!") -> ()  [unwired: 1 in, 1 out]
          }
        }
      }
      event "Execute Leak Test Button": Value Change {
        n131 = event-data() -> ()  [unwired: 1 in, 5 out]
        n132 = flat-sequence {
          tunnel: w193 -> [w196]
          tunnel: [w196] -> w192
          tunnel: w192 -> [w199]
          frame #0 {
            n133 = local write "Test number"(u16 5) -> ()
            n134 = local write "Enum 1"(u16 3 ("Test number")) -> ()
          }
          frame #1 {
            n135 = Enqueue Element(queue=w199, element=Control_3."main" ("Enum")) -> (queue out=w197:refnum<queue>)  [unwired: 2 in, 2 out]
            n136 = Enqueue Element(queue=w197, element=Control_3."start test" ("Enum")) -> ()  [unwired: 2 in, 3 out]
          }
        }
      }
      event "Start Test Button": Value Change {
        n137 = event-data() -> ()  [unwired: 1 in, 5 out]
        n138 = property on="Log Test Button" class="Bool (strict)"() -> ("Value"=w208:bool)  [unwired: 2 in, 2 out]
        n139 = Boolean To (0,1)(Boolean=w208) -> (0, 1=w207:i16)
        n140 = Equal To 0?(x=w207) -> (x = 0?=w206:bool)
        n141 = case shown="True" w206 {
          tunnel: [TRUE ("T button?") w263] -> w201
          frame False {
          }
          frame True {
            # "Log Data Check"
            n142 = Two Button Dialog(message="You are not currently logging data!\nDo you wish to continue?", 1:"No" ("T button name (\"OK\")"), 2:"Yes" ("T button name (\"OK\")")) -> (T button?=w263:bool)
          }
        }
        n143 = Equal?(x=2.0, y=2.0) -> (x = y?=w202:bool)
        n144 = And(x=w202, y=w201) -> (x .and. y?=w203:bool)
        n145 = case shown="True" w203 {
          frame False {
          }
          frame True {
            n146 = flat-sequence {
              tunnel: "Cycle size" -> [w221]
              tunnel: [w221] -> w219
              tunnel: w219 -> [w224]
              tunnel: [w224] -> w218
              tunnel: w218 -> [w227]
              tunnel: [w227] -> w217
              tunnel: w217 -> [w230]
              tunnel: [w230] -> w216
              tunnel: [w233] -> w220
              tunnel: w216 -> [w233]
              tunnel: [w236] -> w215
              tunnel: w220 -> [w236]
              tunnel: w215 -> [w239]
              tunnel: [w239] -> w213
              tunnel: w213 -> [w242]
              tunnel: [w242] -> w212
              tunnel: w212 -> [w245]
              tunnel: [w245] -> w211
              tunnel: w211 -> [w248]
              tunnel: [w248] -> w210
              tunnel: w210 -> [w260]
              frame #0 {
                n147 = call-poly <vilib>:"Read From Spreadsheet File.vi"() -> ("all rows"=w223:dbl[][])  [unwired: 7 in, 4 out]
                n148 = Reshape Array(w223, w221) -> (→"Air Cyc 1":dbl[])
              }
              frame #1 {
                n149 = call-poly <vilib>:"Read From Spreadsheet File.vi"() -> ("all rows"=w225:dbl[][])  [unwired: 7 in, 4 out]
                n150 = Reshape Array(w225, w224) -> (→"Air Cyc 2":dbl[])
              }
              frame #2 {
                n151 = call-poly <vilib>:"Read From Spreadsheet File.vi"() -> ("all rows"=w229:dbl[][])  [unwired: 7 in, 4 out]
                n152 = Reshape Array(w229, w227) -> (→"HC Cyc 1":dbl[])
              }
              frame #3 {
                n153 = call-poly <vilib>:"Read From Spreadsheet File.vi"() -> ("all rows"=w232:dbl[][])  [unwired: 7 in, 4 out]
                n154 = Reshape Array(w232, w230) -> (→"HC Cyc 2":dbl[])
              }
              frame #4 {
                n155 = call-poly <vilib>:"Read From Spreadsheet File.vi"() -> ("all rows"=w234:dbl[][])  [unwired: 7 in, 4 out]
                n156 = Reshape Array(w234, w233) -> (→"Air Bal":dbl[])
              }
              frame #5 {
                n157 = call-poly <vilib>:"Read From Spreadsheet File.vi"() -> ("all rows"=w238:dbl[][])  [unwired: 7 in, 4 out]
                n158 = Reshape Array(w238, w236) -> (→"HC Bal":dbl[])
              }
              frame #6 {
                n159 = call-poly <vilib>:"Read From Spreadsheet File.vi"() -> ("all rows"=w240:dbl[][])  [unwired: 7 in, 4 out]
                n160 = Reshape Array(w240, w239) -> (→"SO Valve 1":dbl[])
              }
              frame #7 {
                n161 = call-poly <vilib>:"Read From Spreadsheet File.vi"() -> ("all rows"=w243:dbl[][])  [unwired: 7 in, 4 out]
                n162 = Reshape Array(w243, w242) -> (→"SO Valve 2":dbl[])
              }
              frame #8 {
                n163 = call-poly <vilib>:"Read From Spreadsheet File.vi"() -> ("all rows"=w247:dbl[][])  [unwired: 7 in, 4 out]
                n164 = Reshape Array(w247, w245) -> (→"Open/Closed \nLoop":dbl[])
              }
              frame #9 {
                n165 = local read "Open/Closed \nLoop"() -> (w249:dbl[])
                n166 = local read "SO Valve 1"() -> (w251:dbl[])
                n167 = local read "SO Valve 2"() -> (w250:dbl[])
                n168 = local read "HC Cyc 2"() -> (w255:dbl[])
                n169 = local read "HC Cyc 1"() -> (w254:dbl[])
                n170 = local read "Air Cyc 1"() -> (w252:dbl[])
                n171 = local read "Air Cyc 2"() -> (w253:dbl[])
                n172 = local read "HC Bal"() -> (w257:dbl[])
                n173 = local read "Air Bal"() -> (w256:dbl[])
                n174 = Build Array (concatenate)(w248, w252, w253, w254, w255, w256, w257, w251, w250, w249) -> (w258:dbl[])
                n175 = shared-variable "My Computer\\Library 1.lvlib\\Inject_Arrays"(w258) -> ()  [unwired: 1 in, 1 out]
              }
              frame #10 {
                n176 = call-poly <vilib>:"Read From Spreadsheet File.vi"() -> ("all rows"=w261:dbl[][])  [unwired: 7 in, 4 out]
                n177 = Reshape Array(w261, w260) -> (w259:dbl[])
                "Lambda" <- w259
                n178 = shared-variable "My Computer\\Library 1.lvlib\\Inject_Arrays_Lambda"(w259) -> ()  [unwired: 1 in, 1 out]
              }
            }
          }
        }
        n179 = case shown="True" w201 {
          tunnel: w209 -> [_ w268]
          frame False {
          }
          frame True {
            n180 = flat-sequence {
              tunnel: w268 -> [w271]
              tunnel: [w271] -> w267
              tunnel: w267 -> [w275]
              frame #0 {
                n181 = local write "Enum 1"(u16 1 ("Test number")) -> ()
                "Test number" <- "Select Test Type"
              }
              frame #1 {
                n182 = Enqueue Element(queue=w275, element=Control_3."main" ("Enum")) -> (queue out=w273:refnum<queue>)  [unwired: 2 in, 2 out]
                n183 = property on="Stop Test Button" class="Bool"("DisabledEnum"=T11."Enabled" ("Disabled")) -> ()  [unwired: 2 in, 2 out]
                n184 = Enqueue Element(queue=w273, element=Control_3."start test" ("Enum")) -> ()  [unwired: 2 in, 3 out]
              }
            }
          }
        }
      }
      event "Log Test Button": Value Change {
        n185 = event-data() -> ()  [unwired: 1 in, 6 out]
        n186 = property on="File Name" class="Str (strict)"() -> ("Value"=w279:T5)  [unwired: 2 in, 2 out]
        n187 = String Length(string=w279) -> (length=w278:i32)
        n188 = Equal To 0?(x=w278) -> (x = 0?=w277:bool)
        n189 = case shown="True" w277 {
          frame False {
          }
          frame True {
            n190 = One Button Dialog(message="A filename has not been entered!") -> ()  [unwired: 1 in, 1 out]
          }
        }
      }
      event "Stop Test Button": Value Change {
        n191 = event-data() -> ()  [unwired: 1 in, 5 out]
        n192 = flat-sequence {
          tunnel: w286 -> [w288]
          tunnel: [w288] -> w285
          tunnel: [w287] -> w283
          tunnel: w285 -> [w292]
          tunnel: [w291] -> w284
          tunnel: w283 -> [w291]
          tunnel: [w290] -> w282
          tunnel: w284 -> [w296]
          tunnel: w282 -> [w295]
          tunnel: [T11."Disabled and Grayed Out" ("Disabled")] -> w281
          frame #0 {
            n193 = local read "Connected?"() -> (w287:bool)
            n194 = local write "Stop Cmd"(T1 1.0 ("Stop Cmd")) -> ()
          }
          frame #1 {
            n195 = Enqueue Element(queue=w292, element=Control_3."main" ("Enum")) -> (queue out=w290:refnum<queue>)  [unwired: 2 in, 2 out]
          }
          frame #2 {
            n196 = case shown="True" w296 {
              tunnel: w295 -> [w297 w300]
              tunnel: [w297 w299] -> _
              frame False {
              }
              frame True {
                n197 = local write "Connected?"(FALSE ("Connected?")) -> ()
                n198 = Enqueue Element(queue=w300, element=Control_3."Multigas disconnect" ("Enum")) -> (queue out=w299:refnum<queue>)  [unwired: 2 in, 2 out]
              }
            }
          }
        }
        n199 = property on="Stop Test Button" class="Bool"("DisabledEnum"=w281) -> ()  [unwired: 2 in, 2 out]
      }
      event "Stopped?": Value Change {
        n200 = event-data() -> ()  [unwired: 1 in, 5 out]
        n201 = flat-sequence {
          tunnel: w304 -> [w308]
          tunnel: [w307] -> w303
          tunnel: [w306] -> w302
          tunnel: w303 -> [w310]
          tunnel: w302 -> [w309]
          frame #0 {
            n202 = local read "Connected?"() -> (w306:bool)
            n203 = Enqueue Element(queue=w308, element=Control_3."main" ("Enum")) -> (queue out=w307:refnum<queue>)  [unwired: 2 in, 2 out]
          }
          frame #1 {
            n204 = case shown="True" w309 {
              tunnel: w310 -> [_ w311]
              frame False {
              }
              frame True {
                n205 = local write "Connected?"(FALSE ("Connected?")) -> ()
                n206 = Enqueue Element(queue=w311, element=Control_3."Multigas disconnect" ("Enum")) -> ()  [unwired: 2 in, 3 out]
              }
            }
          }
        }
      }
      event "Alarm ack": Value Change {
        # "system alarm - set to off"
        n207 = event-data() -> ()  [unwired: 1 in, 5 out]
        n208 = local write "Acknowledge"(TRUE ("Acknowledge")) -> ()
        n209 = property on="Soft Alarm" class="Bool (strict)"("Value"=FALSE ("Acknowledge")) -> ()  [unwired: 2 in, 2 out]
        n210 = property on="Alarm ack" class="Bool"("DisabledEnum"=T11."Disabled and Grayed Out" ("Disabled")) -> ()  [unwired: 2 in, 2 out]
      }
      event "Purge System": Value Change {
        n211 = event-data() -> ()  [unwired: 1 in, 5 out]
        n212 = flat-sequence {
          tunnel: w318 -> [w320]
          tunnel: [w320] -> w317
          tunnel: w317 -> [w321]
          frame #0 {
            n213 = local write "Enum 1"(u16 4 ("Test number")) -> ()
          }
          frame #1 {
            n214 = Enqueue Element(queue=w321, element=Control_3."start test" ("Enum")) -> ()  [unwired: 2 in, 3 out]
          }
        }
      }
      event "Clear log": Value Change {
        n215 = event-data() -> ()  [unwired: 1 in, 5 out]
        n216 = local write "Table"(string[][] [] ("Table")) -> ()
      }
      event "Advanced settings": Value Change {
        # "To be updated"
        # "SO2 conc\nNOx conc\nCO conc\nHC conc\nBleed ratio N2\nBleed ratio CO2"
        n217 = event-data() -> ()  [unwired: 1 in, 5 out]
        n218 = call "Advanced settings MAX.vi"() -> ("output cluster"=→"output cluster":T2)  [unwired: 1 in]
      }
    }
    "stop 2" <- w39
  }
  n219 = node-c288(nitl_modes."Discard missed periods, maintain original phase" ("Mode")) -> (w9:T12)  [unwired: 4 in]
  n220 = node-c288() -> (w2:T12)  [unwired: 4 in]
  n221 = timed-loop {
    timing: w9 -> [_]
    timing-out: [_] -> w8
    shift-right: [w344] -> _
    shift-left: path "" -> [w472]
    shift-right: [w430] -> _
    shift-left: w3 -> [w471]
    shift-right: [w345] -> _
    shift-left: _ -> [w441]
    shift-right: [w420] -> _
    shift-left: w3 -> [w423]
    shift-right: [w421] -> _
    shift-left: w3 -> [w422]
    stop <- w470 stop-if-true
    w354 = 54321.0 ("y")
    # "0   Flow Rate 1\n1   Flow Rate 2\n     ECM 1\n     ECM 2\n2   CO2 U\n3   CO U\n4   HC U\n5   O2 U\n7   CO2 D\n8   CO D\n9   HC D\n10 O2 D\n12 TC1X\n13 TC2A\n14 TC3Y\n15 TC4B\n16 TC5\n17 TC6\n32 Venturi 1\n33 Venturi 2\n34 Tank\n35 Bearing 1\n36 Bearing 2\n38 Ex A\n39 Ex B\n40 Ex C\n41 Ex D\n     MFC Box\n42 Furnace 1\n43 Furnace 2\n44 NO 1 ?? \n45 Lambda 1\n46 NO 2 ??\n47 Lambda 2"
    n222 = node-c288() -> (→"Finished Late? [i-1]":bool, →"Iteration Duration":i64)  [unwired: 1 in, 1 out]
    n223 = shared-variable "My Computer\\Library 1.lvlib\\DATA"() -> (w469:dbl[])  [unwired: 1 in, 1 out]
    n224 = local read "MKS 1"() -> (w364:i16)
    n225 = local read "MKS 2"() -> (w363:i16)
    n226 = case shown="1" w363 {
      tunnel: [dbl[] [54321.0] w582] -> w360
      frame 0, Default {
      }
      frame 1 {
        # "Connecting to MKS Analyser 2"
        n227 = call "tw_PollRequest simple version.vi"("EVID list"=i32[] [2000, 2001, 2002, 2003, 2004, 2005, 2006, 2007, 2008, 2009, 2010, 2011, 2012, 2013, 2014], "IP_ADD [127.0.0.1]"="192.168.254.2") -> ("values out"=w580:string[])  [unwired: 7 in, 2 out]
        n228 = for {
          tunnel: [w584] -> w578 mode=indexing
          tunnel: w580 -> [w583] mode=indexing
          n229 = Fract/Exp String To Number(string=w583) -> (number=w584:dbl)  [unwired: 3 in, 1 out]
        }
        n230 = Build Array (concatenate)(w578) -> (w582:dbl[])
      }
    }
    n231 = case shown="1" w364 {
      tunnel: [dbl[] [54321.0] w586] -> w362
      frame 0, Default {
      }
      frame 1 {
        # "Connecting to MKS Analyser 1"
        n232 = call "tw_PollRequest simple version.vi"("EVID list"=i32[] [2000, 2001, 2002, 2003, 2004, 2005, 2006, 2007, 2008, 2009, 2010, 2011, 2012, 2013, 2014], "IP_ADD [127.0.0.1]"="192.168.254.1") -> ("values out"=w589:string[])  [unwired: 7 in, 2 out]
        n233 = for {
          tunnel: [w592] -> w587 mode=indexing
          tunnel: w589 -> [w591] mode=indexing
          n234 = Fract/Exp String To Number(string=w591) -> (number=w592:dbl)  [unwired: 3 in, 1 out]
        }
        n235 = Build Array (concatenate)(w587) -> (w586:dbl[])
      }
    }
    n236 = Type Cast(type=w469, x=w469) -> (*(type *) &x=w480:dbl[])
    n237 = local read "Advanced Logging"() -> (w350:bool)
    n238 = Delete From Array(array=w480, length=4, index=0) -> (deleted portion=w477:dbl[], array with subset deleted=w327:dbl[])
    n239 = local read "Full system?"() -> (w341:bool)
    n240 = case shown="False" w350 {
      tunnel: [w502 w553] -> w351
      tunnel: w327 -> [w503 w553]
      tunnel: [w501 "Time\tFlow 1 g/s\tFlow 2 g/s\tECM AFR\tCO2 U %\tCO U %\tHC U ppm\tO2 U %\tNO U ppm\tCO2 D %\tCO D %\tHC D ppm\tO2 D %\tNO D ppm\tTC1X\tTC2A\tTCY\tTC4B\tTC5\tTC6\tTC7\tTC8\tTC9\tTC10\tTC11\tTC12\tTC13\tTC14\tTC15\tTC16\tTC17\tTC18\tTC19\tTC20\tTC Vent 1\tTC Vent 2\tTC Tank\tTC Fan B1\tTC Fan B2\tTC Cab\tTC Ex A\tTC Ex B\tTC Ex C\tTC Ex D\tTC MFC Box\tTC Furn 1\tTC Furn 2\tTank Pressure\tRapidox\tLambda 1\tLambda 2\tNOX 1 ppm\tNOX 2 ppm\tUEGO 1\tUEGO 2" ("Heading string 2")] -> w349
      tunnel: w341 -> [w500 _]
      frame False {
        n241 = case shown="True" w500 {
          tunnel: w503 -> [w518 w533]
          tunnel: [w509 w535] -> w502
          tunnel: ["Time\tFlow 1 g/s\tCO2 U %\tCO U %\tHC U ppm\tO2 U %\tNO U ppm\tCO2 D %\tCO D %\tHC D ppm\tO2 D %\tNO D ppm\tTC1X\tTC2A\tTCY\tTC4B\tTC5\tTC6\tTC7\tTC8\tRapidox\tLambda 1\tLambda 2\tNOX 1 ppm\tNOX 2 ppm\tUEGO 1\tUEGO 2" ("Heading string 2") "Time\tFlow 1 g/s\tFlow 2 g/s\tCO2 U %\tCO U %\tHC U ppm\tO2 U %\tNO U ppm\tCO2 D %\tCO D %\tHC D ppm\tO2 D %\tNO D ppm\tTC1X\tTC2A\tTCY\tTC4B\tTC5\tTC6\tTC7\tTC8\tRapidox\tLambda 1\tLambda 2\tNOX 1 ppm\tNOX 2 ppm\tUEGO 1\tUEGO 2" ("Heading string 2")] -> w501
          frame False {
            n242 = Delete From Array(array=w518, length=21, index=0) -> (deleted portion=w505:dbl[], array with subset deleted=w517:dbl[])
            n243 = Index Array(array=w517, index #1=47 ("index"), index #2=48 ("index"), index #3=49 ("index"), index #4=50 ("index"), index #5=51 ("index"), index #6=52 ("index"), index #7=53 ("index")) -> (element #1=w516:dbl, element #2=w515:dbl, element #3=w514:dbl, element #4=w513:dbl, element #5=w512:dbl, element #6=w511:dbl, element #7=w510:dbl)
            n244 = Delete From Array(array=w505, length=1, index=2) -> (array with subset deleted=w504:dbl[])  [unwired: 1 out]
            n245 = Build Array (concatenate)(w504, w516, w515, w514, w513, w512, w511, w510) -> (w509:dbl[])
          }
          frame True {
            n246 = Delete From Array(array=w533, length=21, index=0) -> (deleted portion=w530:dbl[], array with subset deleted=w534:dbl[])
            n247 = Index Array(array=w534, index #1=47 ("index"), index #2=48 ("index"), index #3=49 ("index"), index #4=50 ("index"), index #5=51 ("index"), index #6=52 ("index"), index #7=53 ("index")) -> (element #1=w542:dbl, element #2=w541:dbl, element #3=w540:dbl, element #4=w539:dbl, element #5=w538:dbl, element #6=w537:dbl, element #7=w536:dbl)
            n248 = Delete From Array(array=w530, length=2, index=1) -> (array with subset deleted=w528:dbl[])  [unwired: 1 out]
            n249 = Build Array (concatenate)(w528, w542, w541, w540, w539, w538, w537, w536) -> (w535:dbl[])
          }
        }
      }
      frame True {
        (unwired) "Time\tFlow 1 g/s\tFlow 2 g/s\tECM AFR\tCO2 U %\tCO U %\tHC U ppm\tO2 U %\tNO U ppm\tCO2 D %\tCO D %\tHC D ppm\tO2 D %\tNO D ppm\tTC1X\tTC2A\tTCY\tTC4B\tTC5\tTC6\tTC7\tTC8\tTC9\tTC10\tTC11\tTC12\tTC13\tTC14\tTC15\tTC16\tTC17\tTC18\tTC19\tTC20\tTC Vent 1\tTC Vent 2\tTC Fan B1\tTC Fan B2\tTC Cab\tTC Ex A\tTC Ex B\tTC Ex C\tTC Ex D\tTC Furn 1\tTC Furn 2\tNOX 1 ppm\tNLambda 1\tNOX 2 ppm\tNLambda 2\tEGO 1\tEGO 2\tEGO 3\tEGO 4\tCO2 U %\tCO U %\tHC U ppm\tO2 U %\tNO U ppm\tCO2 D %\tCO D %\tHC D ppm\tO2 D %\tNO D ppm\r\n" ("Heading string 2")
      }
    }
    n250 = Index Array(array=w477) -> (element #1=w345:dbl, element #2=w447:dbl, element #3=w347:dbl, element #4=w440:dbl)  [unwired: 4 in]
    "Error" <- w347
    n251 = To Unsigned Long Integer(number=w440) -> (unsigned 32bit integer=w439:u32)
    n252 = Number To Boolean Array(number=w439) -> (Boolean array=w459:bool[])
    n253 = Index Array(array=w459) -> (element #2=w457:bool, element #3=w456:bool, element #4=w436:bool, element #5=→"ExtAnUp":bool, element #6=→"ExtAnDn":bool)  [unwired: 6 in, 1 out]
    "Extractor Fan On" <- w436
    n254 = case shown="2" w447 {
      tunnel: [w612 TRUE FALSE] -> w446
      tunnel: [w613 FALSE TRUE] -> w445
      frame 0, Default {
        n255 = local read "Pass"() -> (w613:bool)
        n256 = local read "Fail"() -> (w612:bool)
      }
      frame 1 {
      }
      frame 2 {
      }
    }
    "Pass" <- w445
    "Fail" <- w446
    n257 = Or(x=w457, y=w456) -> (x .or. y?=→"Doors Open":bool)
    n258 = Not(x=w436) -> (.not. x?=→"Doors Unlocked":bool)
    n259 = Less?(x=w345, y=w441) -> (x < y?=w438:bool)
    n260 = Path To String(path="File Path") -> (string=w434:string)
    n261 = Index Array(array=w362, index=0) -> (element=w358:dbl)
    n262 = Index Array(array=w360, index=0) -> (element=w356:dbl)
    n263 = local read "Connected"() -> (w437:bool)
    n264 = Concatenate Strings(w434, "\\" ("string"), "File Name") -> (w365:string)
    n265 = Not Equal?(x=w358, y=w354) -> (x != y?=w357:bool)
    n266 = Not Equal?(x=w354, y=w356) -> (x != y?=w355:bool)
    n267 = case shown="True" w357 {
      tunnel: [w559 w570] -> w353
      tunnel: w360 -> [w558 w569]
      tunnel: w362 -> [_ w568]
      tunnel: w355 -> [w557 w567]
      tunnel: [w556 w564] -> w352
      frame False {
        n268 = case shown="False" w557 {
          tunnel: [dbl[] [54321.0] w563] -> w559
          tunnel: w558 -> [_ w563]
          tunnel: ["\r\n" ("Heading string 2") "\tNO\tNO2 (150)\tNO2 (2000)\tN2O\tNH3 (300)\tNH3 (3000)\tHNCO (400)\tH2O\tCO2\tCO (500)\tCO (1)\tCH4 (250)\tCH4 (3000)\tNOxP\tPropane\r\n" ("Heading string 2")] -> w554
          frame False {
          }
          frame True {
          }
        }
        n269 = Build Array(" " ("Heading string 2"), w554) -> (w556:string[])
      }
      frame True {
        n270 = case shown="True" w567 {
          tunnel: [w572 w576] -> w570
          tunnel: w569 -> [_ w575]
          tunnel: w568 -> [w572 w574]
          tunnel: ["\rn" ("Heading string 2") "\tNO\tNO2 (150)\tNO2 (2000)\tN2O\tNH3 (300)\tNH3 (3000)\tHNCO (400)\tH2O\tCO2\tCO (500)\tCO (1)\tCH4 (250)\tCH4 (3000)\tNOxP\tPropane\r" ("Heading string 2")] -> w565
          frame False {
          }
          frame True {
            n271 = Build Array (concatenate)(w574, w575) -> (w576:dbl[])
          }
        }
        n272 = Build Array("\tNO\tNO2 (150)\tNO2 (2000)\tN2O\tNH3 (300)\tNH3 (3000)\tHNCO (400)\tH2O\tCO2\tCO (500)\tCO (1)\tCH4 (250)\tCH4 (3000)\tNOxP\tPropane" ("Heading string 2"), w565) -> (w564:string[])
      }
    }
    n273 = And(x=w437, y=w438) -> (x .and. y?=w429:bool)
    n274 = local write "Stopped?"(w429) -> ()
    n275 = Equal To 0?(x=w347) -> (x = 0?=w348:bool)
    n276 = Equal To 0?(x=w345) -> (x = 0?=w346:bool)
    n277 = Build Array (concatenate)(w351, w353) -> (w473:dbl[])
    n278 = Equal?(x=w345, y=2.0) -> (x = y?=w373:bool)
    n279 = String To Path(string=w365) -> (path=w431:path)
    n280 = Build Array(w348, w346) -> (w453:bool[])
    n281 = Equal?(x=w345, y=3.0) -> (x = y?=w370:bool)
    n282 = Equal?(x=w345, y=4.0) -> (x = y?=w368:bool)
    n283 = Boolean Array To Number(Boolean array=w453) -> (number=w452:u32)
    n284 = Not Equal?(x=w431, y=w472) -> (x != y?=w482:bool)
    n285 = Compound Arithmetic op=OR(w373, w370, w368) -> (w372:bool)
    n286 = local read "Log Test Button"() -> (w366:bool)
    n287 = case shown="2" w452 {
      tunnel: [w637 w638 w643 w645] -> w454
      tunnel: [w637 w638 w643 w645] -> w451
      tunnel: [w637 w638 w643 w645] -> w450
      tunnel: [w637 w638 w641 w645] -> w449
      tunnel: [T11."Enabled" ("Disabled") T11."Enabled" ("Disabled") w641 w645] -> w448
      tunnel: [FALSE FALSE FALSE TRUE] -> w428
      frame 0, Default {
        w637 = T11."Disabled and Grayed Out" ("Disabled")
      }
      frame 1 {
        w638 = T11."Disabled and Grayed Out" ("Disabled")
      }
      frame 2 {
        w641 = T11."Enabled" ("Disabled")
        w643 = T11."Disabled and Grayed Out" ("Disabled")
      }
      frame 3 {
        w645 = T11."Enabled" ("Disabled")
        (unwired) T11."Disabled and Grayed Out" ("Disabled")
      }
    }
    n288 = for {
      tunnel: w473 -> [w653] mode=indexing
      tunnel: [w652] -> w484 mode=indexing
      n289 = Number To Fractional String(number=w653, precision (6)=i16 3) -> (F-format string=w652:string)  [unwired: 2 in]
    }
    n290 = Select(t=w431, s=w482, f=w472) -> (s? t:f=w483:path)
    n291 = And(x=w366, y=w372) -> (x .and. y?=w499:bool)
    "Log?" <- w499
    n292 = case shown="True" w482 {
      tunnel: w483 -> [w646 w651]
      tunnel: [w646 w650] -> w481
      tunnel: w352 -> [_ w648]
      tunnel: w349 -> [_ w647]
      frame False {
      }
      frame True {
        # "setting up the header"
        n293 = Build Array (concatenate)(w647, w648) -> (w649:string[])
        n294 = call-poly <vilib>:"Write To Spreadsheet File.vi"("1D data"=w649, "file path (dialog if empty)"=w651) -> ("new file path (Not A Path if cancelled)"=w650:path)  [unwired: 6 in]
      }
    }
    n295 = Equal?(x=w345, y=0.0) -> (x = y?=w417:bool)
    n296 = case shown="5" w345 {
      tunnel: [w599 w602 w604 w606 TRUE FALSE] -> w444
      tunnel: [w599 TRUE TRUE TRUE w608 w610] -> w443
      tunnel: [TRUE w602 w604 w606 w608 w610] -> w442
      frame 0, Default {
        w599 = FALSE
      }
      frame 1 {
        w602 = FALSE
      }
      frame 2 {
        w604 = FALSE
      }
      frame 3 {
        w606 = FALSE
      }
      frame 4 {
        w608 = FALSE
        n297 = local write "Stop Cmd"(T1 0.0 ("Stop Cmd")) -> ()
      }
      frame 5 {
        w610 = FALSE
      }
    }
    "Cool Down" <- w444
    "Test In Progress" <- w443
    "Standby" <- w442
    n298 = property class="VI"("Front Panel.Closeable"=w428) -> ()  [unwired: 2 in, 2 out]
    n299 = property on="Start Test Button" class="Bool"("DisabledEnum"=w454) -> ()  [unwired: 2 in, 2 out]
    n300 = property on="Execute Leak Test Button" class="Bool"("DisabledEnum"=w451) -> ()  [unwired: 2 in, 2 out]
    n301 = property on="Compile Test Button" class="Bool"("DisabledEnum"=w450) -> ()  [unwired: 2 in, 2 out]
    n302 = property on="Purge System" class="Bool"("DisabledEnum"=w449) -> ()  [unwired: 2 in, 2 out]
    n303 = property on="Advanced settings" class="Bool"("DisabledEnum"=w448) -> ()  [unwired: 2 in, 2 out]
    n304 = Index Array(array=w353, index #1=0 ("index"), index #2=1 ("index"), index #3=2 ("index"), index #4=3 ("index")) -> ()  [unwired: 4 out]
    n305 = local read "Full system?"() -> (w418:bool)
    n306 = Not Equal To 0?(x=w347) -> (x != 0?=w475:bool)
    n307 = Not Equal?(x=w347, y=w471) -> (x != y?=w474:bool)
    n308 = case shown="True" w499 {
      tunnel: w481 -> [w657 w665]
      tunnel: [w657 w677] -> w344
      tunnel: w484 -> [_ w673]
      tunnel: w423 -> [_ w666]
      tunnel: w422 -> [w656 w661]
      tunnel: [w656 w663] -> w421
      tunnel: [w655 w662] -> w420
      frame False {
        n309 = local read "Log interval (seconds)"() -> (w655:T1)
      }
      frame True {
        n310 = Get Date/Time In Seconds() -> (seconds since 1Jan1904=w674:timestamp)
        n311 = Decrement(x=w666) -> (x-1=w667:T1)
        n312 = Less Than 0?(x=w667) -> (x < 0?=w668:bool)
        n313 = Equal To 0?(x=w667) -> (x = 0?=w669:bool)
        n314 = Build Array(w668, w669) -> (w670:bool[])
        n315 = Path To String(path=w665) -> (string=w660:string)
        "File name" <- w660
        n316 = Format Date/Time String(time format string (%c)="%d/%m/%y %H:%M:%S", seconds (now)=w674) -> (date/time string=w675:string)  [unwired: 1 in]
        n317 = Boolean Array To Number(Boolean array=w670) -> (number=w671:u32)
        n318 = case shown="2" w671 {
          tunnel: w666 -> [w684 w685 _]
          tunnel: [w683 w685 w688] -> w662
          tunnel: w660 -> [w682 w687 w691]
          tunnel: [w679 w687 w689] -> w664
          tunnel: [w678 w686 w690] -> w663
          tunnel: w661 -> [w678 w686 w694]
          frame 0, Default {
            n319 = Number To Decimal String(number=w678) -> (decimal integer string=w680:string)  [unwired: 1 in]
            n320 = call <vilib>:"Space Constant.vi"() -> ("String"=w681:string)
            n321 = Decrement(x=w684) -> (x-1=w683:T1)
            n322 = Concatenate Strings(w682, w681, w680) -> (w679:string)
          }
          frame 1 {
          }
          frame 2 {
            n323 = Increment(x=w694) -> (x+1=w690:dbl)
            n324 = local read "Log interval (seconds)"() -> (w688:T1)
            n325 = Number To Decimal String(number=w690) -> (decimal integer string=w692:string)  [unwired: 1 in]
            n326 = call <vilib>:"Space Constant.vi"() -> ("String"=w693:string)
            n327 = Concatenate Strings(w691, w693, w692) -> (w689:string)
          }
        }
        n328 = Build Array (concatenate)(w675, w673) -> (w659:string[])
        n329 = String To Path(string=w664) -> (path=w658:path)
        n330 = call-poly <vilib>:"Write To Spreadsheet File.vi"("append to file? (new file:F)"=TRUE, "1D data"=w659, "file path (dialog if empty)"=w658) -> ("new file path (Not A Path if cancelled)"=w677:path)  [unwired: 5 in]
      }
    }
    n331 = And(x=w475, y=w474) -> (x .and. y?=w476:bool)
    n332 = Index Array(array=w327, index #1=0 ("index"), index #2=1 ("index"), index #3=4 ("index"), index #4=5 ("index"), index #5=7 ("index"), index #6=9 ("index"), index #7=10 ("index"), index #8=12 ("index"), index #9=6 ("index"), index #10=11 ("index"), index #11=14 ("index"), index #12=15 ("index"), index #13=16 ("index"), index #14=17 ("index"), index #15=18 ("index"), index #16=19 ("index"), index #17=34 ("index"), index #18=35 ("index"), index #19=36 ("index"), index #20=37 ("index"), index #21=38 ("index"), index #22=40 ("index"), index #23=41 ("index"), index #24=42 ("index"), index #25=43 ("index"), index #26=45 ("index"), index #27=46 ("index"), index #28=51 ("index"), index #29=52 ("index"), index #30=49 ("index"), index #31=50 ("index"), index #32=2 ("index"), index #33=3 ("index")) -> (element #1=w326:dbl, element #2=w325:dbl, element #3=w413:dbl, element #4=w412:dbl, element #5=w340:dbl, element #6=w339:dbl, element #7=w338:dbl, element #8=w337:dbl, element #9=w336:dbl, element #10=w335:dbl, element #11=w407:dbl, element #12=w406:dbl, element #13=w405:dbl, element #14=w404:dbl, element #15=w403:dbl, element #16=w402:dbl, element #17=w396:dbl, element #18=w395:dbl, element #19=w394:dbl, element #20=w393:dbl, element #21=w392:dbl, element #22=w387:dbl, element #23=w386:dbl, element #24=w385:dbl, element #25=w384:dbl, element #26=→"Furnace temp 1":dbl, element #27=→"Furnace temp 2":dbl, element #28=w377:dbl, element #29=w343:dbl, element #30=w342:dbl, element #31=w374:dbl, element #32=w329:dbl, element #33=w328:dbl)
    n333 = Build Array(w418, w417) -> (w419:bool[])
    n334 = case shown="True" w476 {
      tunnel: w347 -> [w619 w630]
      tunnel: w474 -> [w622 _]
      tunnel: [w618 w630] -> w430
      frame False {
        n335 = Equal To 0?(x=w619) -> (x = 0?=w623:bool)
        n336 = And(x=w623, y=w622) -> (x .and. y?=w621:bool)
        n337 = case shown="True" w621 {
          frame False {
          }
          frame True {
            w626 = FALSE ("Ack hard alarm!")
            n338 = property on="Hard Alarm" class="Bool (strict)"("Value"=w626) -> ()  [unwired: 2 in, 2 out]
            n339 = property on="System Alarm" class="Bool (strict)"("Value"=w626) -> ()  [unwired: 2 in, 2 out]
          }
        }
        n340 = case shown="False" "Acknowledge" {
          tunnel: [w624 0.0 ("Numeric")] -> w618
          tunnel: w619 -> [w624 _]
          frame False {
          }
          frame True {
          }
        }
      }
      frame True {
        n341 = local read "Table"() -> (w633:string[][])
        n342 = call "Error list.vi"("Error code"=w630, "Error array in"=w633) -> ("Hard alarm?"=w627:bool, "Error array out"=w632:string[][])  [unwired: 8 in]
        "Hard Alarm" <- w627
        "System Alarm" <- w627
        n343 = Not(x=w627) -> (.not. x?=w628:bool)
        "Soft Alarm" <- w628
        n344 = case shown="True" w628 {
          frame False {
          }
          frame True {
            n345 = property on="Alarm ack" class="Bool"("DisabledEnum"=T11."Enabled" ("Disabled")) -> ()  [unwired: 2 in, 2 out]
          }
        }
        n346 = local write "Table"(w632) -> ()
        n347 = local write "Acknowledge"(FALSE ("Acknowledge")) -> ()
        n348 = property on="Tab Control" class="TabCtl (strict)"("Value"=6) -> ()  [unwired: 2 in, 2 out]
      }
    }
    n349 = Boolean Array To Number(Boolean array=w419) -> (number=w416:u32)
    n350 = case shown="1" w416 {
      tunnel: w326 -> [w594 w596 _ _]
      tunnel: w325 -> [_ w595 _ _]
      tunnel: [w594 w596 w597 w598] -> w415
      tunnel: [0.0 ("y") w595 w597 w598] -> w414
      frame 0, Default {
      }
      frame 1 {
      }
      frame 2 {
        w597 = 0.0 ("y")
      }
      frame 3 {
        w598 = 0.0 ("y")
      }
    }
    n351 = Merge Signals(w415, w414) -> (→"Flow Rate (g/s)":dynamicdata)
    n352 = Merge Signals(w413, w412, w340, w339, w338, w337) -> (→"M584L Upstream & Downstream":dynamicdata)
    n353 = Merge Signals(w407, w406, w405, w404, w403, w402) -> (→"Sample Temperatures (°C)":dynamicdata)
    n354 = Merge Signals(w396, w395, w394, w393, w392) -> (→"System Temperatures (°C)":dynamicdata)
    n355 = Merge Signals(w387, w386, w385, w384) -> (→"Heat Exchanger Temperatures (°C)":dynamicdata)
    n356 = Merge Signals(w377, w343) -> (→"NO Concentration (ppm)":dynamicdata)
    n357 = Merge Signals(w342, w374, w329, w328) -> (→"Lambda":dynamicdata)
    n358 = local read "MKS HC"() -> (w332:dbl)
    n359 = Merge Signals(w336, w335, w332) -> (→"HC Concentration (ppm)":dynamicdata)
    n360 = local read "stop 2"() -> (w470:bool)
    n361 = node-c288() -> ()  [unwired: 1 in, 1 out]
  }
  n362 = timed-loop {
    timing: w2 -> [_]
    timing-out: [_] -> w1
    stop <- _ stop-if-true
    n363 = node-c288() -> ()  [unwired: 1 in, 1 out]
    n364 = shared-variable "My Computer\\Library 1.lvlib\\DATA_2"() -> (w703:dbl[])  [unwired: 1 in, 1 out]
    n365 = case shown="True" "MKS" {
      tunnel: [dbl[] [] w724] -> w701
      frame False {
      }
      frame True {
        # "Connecting to MKS Analyser 2"
        n366 = call "tw_PollRequest simple version.vi"("EVID list"=i32[] [2000, 2001, 2002, 2003, 2004, 2005, 2006, 2007, 2008, 2009, 2010, 2011, 2012, 2013, 2014, 2015, 2016, 2017], "IP_ADD [127.0.0.1]"="192.168.254.2") -> ("values out"=w726:string[])  [unwired: 7 in, 2 out]
        n367 = for {
          tunnel: [w730] -> w728 mode=indexing
          tunnel: w726 -> [w729] mode=indexing
          n368 = Fract/Exp String To Number(string=w729) -> (number=w730:dbl)  [unwired: 3 in, 1 out]
        }
        n369 = Build Array (concatenate)(w728) -> (w724:dbl[])
        n370 = Index Array(array=w724, index="HC Index") -> (element=→"MKS HC":dbl)
      }
    }
    n371 = Build Array (concatenate)(w703, w701) -> (w702:dbl[])
    n372 = for {
      tunnel: w702 -> [w737] mode=indexing
      tunnel: [w736] -> w713 mode=indexing
      n373 = Number To Fractional String(number=w737, precision (6)=i16 3) -> (F-format string=w736:string)  [unwired: 2 in]
    }
    n374 = Add(x=0 ("index"), y="MFC Number") -> (x+y=w705:i32)
    n375 = Add(x="MFC Number", y=6) -> (x+y=w704:i32)
    n376 = Index Array(array=w703, index #1=w705, index #2=w704) -> (element #1=w710:dbl, element #2=w709:dbl)
    n377 = Get Date/Time In Seconds() -> (seconds since 1Jan1904=w716:timestamp)
    n378 = local read "File name"() -> (w720:string)
    n379 = Format Date/Time String(time format string (%c)="%d/%m/%y %H:%M:%S", seconds (now)=w716) -> (date/time string=w714:string)  [unwired: 1 in]
    n380 = Concatenate Strings(w720, "_MFC" ("string")) -> (w718:string)
    n381 = Build Array (concatenate)(w714, w713) -> (w712:string[])
    n382 = String To Path(string=w718) -> (path=w715:path)
    n383 = local read "Log?"() -> (w711:bool)
    n384 = case shown="True" w711 {
      tunnel: w715 -> [w731 w734]
      tunnel: [w731 w732] -> _
      tunnel: w712 -> [_ w733]
      frame False {
      }
      frame True {
        n385 = call-poly <vilib>:"Write To Spreadsheet File.vi"("append to file? (new file:F)"=TRUE, "1D data"=w733, "file path (dialog if empty)"=w734) -> ("new file path (Not A Path if cancelled)"=w732:path)  [unwired: 5 in]
      }
    }
    n386 = Merge Signals(w710, w709) -> (→"MFC Setpoint/Delivery":dynamicdata)
    n387 = node-c288() -> ()  [unwired: 1 in, 1 out]
  }
  n388 = while {
    tunnel: w37 -> [w745]
    tunnel: w21 -> [w743]
    tunnel: w23 -> [w742]
    tunnel: [FALSE ("stop 2")] -> w11
    stop <- w746 stop-if-true
    n389 = Dequeue Element(queue=w745) -> (element=w744:T10)  [unwired: 2 in, 3 out]
    n390 = case shown="\"main\", Default" w744 {
      tunnel: w743 -> [_ _ _ w801 w812 w848 w882 _ _ _ _ _ _ _ w1245 _ _ _ _ _ _ _]
      tunnel: w742 -> [_ _ _ _ _ _ _ _ w895 w910 w965 w1010 _ _ _ _ _ _ _ _ _ _]
      frame "main", Default {
        # "20"
        # "25"
        # "30"
        # "15"
        # "10"
        # "5"
        # "0"
        # "30"
        # "25"
        # "20"
        # "15"
        # "10"
        # "5"
        # "0"
        # "Output Cluster\n\n0 NOx Conc\n1 CO conc %\n2 HC conc %\n3 Bleed H2O \n4 Bleed CO2\n5 Bleed N2 \n6 lambda P\n7 lambda I\n8 lambda D\n9 purge duration\n10 Target furnace lambda\n11 HC reaction ct\n12 Full system\n13 Log interval\n14 MKS 1\n15 MKS 2"
        n391 = local read "output cluster"() -> (w775:T2)
        n392 = Unbundle(w775) -> ("NOx Concentration (ppm)"=w761:T1, "CO concentration %"=w760:T1, "HC concentration %"=w759:T1, "Bleed H2O %"=w758:T1, "Bleed CO2 %"=w757:T1, "Bleed N2 %"=w772:T1, "lambda P"=w771:T1, "lambda I"=w770:T1, "lambda D"=w773:T1, "Purge duration (seconds)"=w774:T1, "Target furnace lambda"=w766:T1, "HC reaction constant"=w765:T1, w767:i16, "Log interval (HRS)"=→"Log interval (seconds)":T1, w754:i16, w752:i16, "Advanced Logging"=→"Advanced Logging":bool, "Cycle Length (Hours)"=w750:T1, "Heat Load Control"=w748:bool, w749:T1[])
        "MKS 1" <- w754
        "MKS 2" <- w752
        n393 = local read "Test Flow Rate(g/s)"() -> (w787:T1)
        n394 = local read "Test number"() -> (w792:u16)
        n395 = local read "Inlet LAMBDA"() -> (w779:T1)
        n396 = local read "NO ppm Loff"() -> (w777:T1)
        n397 = local read "NO:CO Ratio"() -> (w776:T1)
        n398 = local read "Inlet O2 (%)"() -> (w778:T1)
        n399 = local read "Connected"() -> (w781:bool)
        n400 = Boolean To (0,1)(Boolean=w748) -> (0, 1=w747:i16)
        n401 = Boolean To (0,1)(Boolean=w781) -> (0, 1=w764:i16)
        n402 = Build Array (concatenate)("Stop Cmd", w792, w787, "Test Start Temperature (°C)", "Test Stop temperature (°C)", "Furnace Ramp Rate (°C/min)", w779, w778, "Inlet LAMBDA Rich", "Inlet LAMBDA Lean", "Inlet Temperature (°C)", "NO ppm SW", w777, w776, "Temperature Limit (°C)", w764, "Inlet temp Age", "Flow rate Age", w761, w760, w759, w758, w757, w772, w771, w770, w773, w774, w766, w765, w767, w750, w747, w749) -> (w783:T1[])
        n403 = Not Equal To 0?(x=w767) -> (x != 0?=→"Full system?":bool)
        n404 = shared-variable "My Computer\\Library 1.lvlib\\Control Variables"(w783) -> ()  [unwired: 1 in, 1 out]
        n405 = Not Equal To 0?(x=w754) -> (x != 0?=w755:bool)
        n406 = Not Equal To 0?(x=w752) -> (x != 0?=w753:bool)
        n407 = Or(x=w755, y=w753) -> (x .or. y?=→"Connected":bool)
      }
      frame "start test" {
        w793 = FALSE
        n408 = property on="Pass" class="Bool (strict)"("Value"=w793) -> ()  [unwired: 2 in, 2 out]
        n409 = property on="Fail" class="Bool (strict)"("Value"=w793) -> ()  [unwired: 2 in, 2 out]
        n410 = local write "Pass"(w793) -> ()
        n411 = local write "Fail"(w793) -> ()
        n412 = shared-variable "My Computer\\Library 1.lvlib\\Enum 1"("Enum 1") -> ()  [unwired: 1 in, 1 out]
      }
      frame "clear table 1" {
        n413 = property on="Sub-Cycle Name" class="Str (strict)"("Value"="" ("Subcycle name")) -> ()  [unwired: 2 in, 2 out]
        n414 = local write "Sub-Cycle Pattern"(string[][] [["", "0", "", "", "", "", "", "", "", "", "", "", ""], ["", "", "", "", "", "", "", "", "", "", "", "", ""], ["", "", "", "", "", "", "", "", "", "", "", "", ""], ["", "", "", "", "", "", "", "", "", "", "", "", ""], ["", "", "", "", "", "", "", "", "", "", "", "", ""], ["", "", "", "", "", "", "", "", "", "", "", "", ""], ["", "", "", "", "", "", "", "", "", "", "", "", ""], ["", "", "", "", "", "", "", "", "", "", "", "", ""], ["", "", "", "", "", "", "", "", "", "", "", "", ""], ["", "", "", "", "", "", "", "", "", "", "", "", ""], ["", "", "", "", "", "", "", "", "", "", "", "", ""], ["", "", "", "", "", "", "", "", "", "", "", "", ""], ["", "", "", "", "", "", "", "", "", "", "", "", ""], ["", "", "", "", "", "", "", "", "", "", "", "", ""], ["", "", "", "", "", "", "", "", "", "", "", "", ""], ["", "", "", "", "", "", "", "", "", "", "", "", ""], ["", "", "", "", "", "", "", "", "", "", "", "", ""], ["", "", "", "", "", "", "", "", "", "", "", "", ""], ["", "", "", "", "", "", "", "", "", "", "", "", ""], ["", "", "", "", "", "", "", "", "", "", "", "", ""], ["", "", "", "", "", "", "", "", "", "", "", "", ""], ["", "", "", "", "", "", "", "", "", "", "", "", ""], ["", "", "", "", "", "", "", "", "", "", "", "", ""], ["", "", "", "", "", "", "", "", "", "", "", "", ""], ["", "", "", "", "", "", "", "", "", "", "", "", ""], ["", "", "", "", "", "", "", "", "", "", "", "", ""], ["", "", "", "", "", "", "", "", "", "", "", "", ""], ["", "", "", "", "", "", "", "", "", "", "", "", ""], ["", "", "", "", "", "", "", "", "", "", "", "", ""], ["", "", "", "", "", "", "", "", "", "", "", "", ""], ["", "", "", "", "", "", "", "", "", "", "", "", ""]]) -> ()
        n415 = local write "Flag1"(FALSE) -> ()
      }
      frame "update list 1" {
        n416 = String To Path(string=w801) -> (path=w800:path)
        n417 = List Folder(path=w800, pattern="*.eyes") -> (filenames=w799:string[])  [unwired: 2 in, 3 out]
        n418 = property on="Sub-Cycle List" class="LstBox (strict)"("Item Names"=w799) -> ()  [unwired: 2 in, 2 out]
      }
      frame "save subc" {
        w805 = ".eyes" ("string")
        n419 = local read "Sub-Cycle Name"() -> (w804:T5)
        n420 = String To Path(string=w812) -> (path=w817:path)
        n421 = Equal?(x=w804, y="") -> (x = y?=w809:bool)
        n422 = List Folder(path=w817, pattern="*.eyes" ("string")) -> (filenames=w816:string[])  [unwired: 2 in, 3 out]
        n423 = Concatenate Strings(w804, w805) -> (w803:string)
        n424 = Concatenate Strings(w812, w804, w805) -> (w818:string)
        n425 = Search 1D Array(1D array=w816, element=w803) -> (index of element=w815:i32)  [unwired: 1 in]
        n426 = case shown="True" w809 {
          tunnel: [TRUE FALSE] -> w808
          frame False {
          }
          frame True {
            n427 = One Button Dialog(message="Insert file name!") -> ()  [unwired: 1 in, 1 out]
          }
        }
        n428 = String To Path(string=w818) -> (path=w811:path)
        n429 = Equal?(x=w815, y=-1) -> (x = y?=w813:bool)
        n430 = case shown="False" w813 {
          selector: w813 -> [_ w824]
          tunnel: [w822 w824] -> w807
          frame False {
            n431 = Two Button Dialog(message="A file with this name already exists!\nDo you want to overwrite?") -> (T button?=w822:bool)  [unwired: 2 in]
          }
          frame True {
          }
        }
        n432 = And(x=w807, y=w808) -> (x .and. y?=w806:bool)
        n433 = case shown="True" w806 {
          tunnel: w811 -> [_ w829]
          frame False {
          }
          frame True {
            n434 = local read "Sub-Cycle Pattern"() -> (w828:string[][])
            n435 = call "Table check.vi"("Input table"=w828) -> ("Incomplete?"=w826:bool, "Length"=w827:i32)  [unwired: 9 in]
            n436 = case shown="False" w826 {
              tunnel: w828 -> [w837 _]
              tunnel: w829 -> [w836 _]
              tunnel: w827 -> [w835 _]
              tunnel: string[] [] -> [w834 _]
              frame False {
                n437 = for {
                  N: w835 -> [_]
                  tunnel: w837 -> [w844]
                  shift-right: [w841] -> w833
                  shift-left: w834 -> [w842]
                  i -> [w843]
                  n438 = Index Array(array=w844, index (row)=w843) -> (element=w840:string[])  [unwired: 1 in]
                  n439 = Delete From Array(array=w840, index=0) -> (array with subset deleted=w839:string[])  [unwired: 1 in, 1 out]
                  n440 = Build Array (concatenate)(w842, w839) -> (w841:string[])
                }
                n441 = Build Array (concatenate)("SubCycle Data File for EYECAT - do not modify", w833) -> (w831:string[])
                n442 = call-poly <vilib>:"Write To Spreadsheet File.vi"("1D data"=w831, "file path (dialog if empty)"=w836) -> ()  [unwired: 6 in, 1 out]
              }
              frame True {
                n443 = One Button Dialog(message="The table is incomplete!\nplease review and save again!") -> ()  [unwired: 1 in, 1 out]
              }
            }
            n444 = local write "Flag1"(FALSE) -> ()
          }
        }
      }
      frame "load subc" {
        n445 = local read "Flag1"() -> (w849:bool)
        n446 = case shown="True" w849 {
          tunnel: [w876 w878] -> w847
          tunnel: w848 -> [w876 w878]
          tunnel: [TRUE w877] -> w846
          frame False {
          }
          frame True {
            n447 = Two Button Dialog(message="The table has been modified.\nDo you want to continue?") -> (T button?=w877:bool)  [unwired: 2 in]
          }
        }
        n448 = case shown="True" w846 {
          tunnel: w847 -> [_ w853]
          frame False {
          }
          frame True {
            n449 = property on="Sub-Cycle List" class="LstBox (strict)"() -> ("Item Names"=w865:string[])  [unwired: 2 in, 2 out]
            n450 = Index Array(array=w865, index="Sub-Cycle List") -> (element=w852:string)
            n451 = Concatenate Strings(w853, w852) -> (w863:string)
            n452 = Search/Split String(string=w852, search string/char (-)=".") -> (substring before match=w850:string)  [unwired: 1 in, 2 out]
            n453 = local write "Sub-Cycle Name"(w850) -> ()
            n454 = String To Path(string=w863) -> (path=w862:path)
            n455 = call-poly <vilib>:"Read From Spreadsheet File.vi"("file path (dialog if empty)"=w862) -> ("first row"=w858:string[])  [unwired: 6 in, 4 out]
            n456 = Delete From Array(array=w858, length=1, index=0) -> (array with subset deleted=w855:string[])  [unwired: 1 out]
            n457 = Array Size(array=w855) -> (size(s)=w861:i32)
            n458 = Divide(x=w861, y=12) -> (x/y=w854:dbl)
            n459 = for {
              N: w854 -> [_]
              shift-right: [w871] -> _
              shift-left: w855 -> [w874]
              tunnel: [w870] -> w859 mode=indexing
              i -> [w869]
              n460 = Increment(x=w869) -> (x+1=w868:i32)
              n461 = Delete From Array(array=w874, length=12, index=0) -> (deleted portion=w866:string[], array with subset deleted=w871:string[])
              n462 = Number To Decimal String(number=w868) -> (decimal integer string=w867:string)  [unwired: 1 in]
              n463 = Build Array (concatenate)(w867, w866) -> (w870:string[])
            }
            n464 = local write "Sub-Cycle Pattern"(w859) -> ()
          }
        }
      }
      frame "delete subc" {
        n465 = Two Button Dialog(message="This operation will permanently delete this file!\nDo you want to continue?") -> (T button?=w881:bool)  [unwired: 2 in]
        n466 = case shown="True" w881 {
          tunnel: w882 -> [_ w887]
          frame False {
          }
          frame True {
            n467 = local read "Sub-Cycle List"() -> (w884:i32)
            n468 = property on="Sub-Cycle List" class="LstBox (strict)"() -> ("Item Names"=w885:string[])  [unwired: 2 in, 2 out]
            n469 = Index Array(array=w885, index=w884) -> (element=w889:string)
            n470 = Concatenate Strings(w887, w889) -> (w888:string)
            n471 = local write "Flag1"(FALSE) -> ()
            n472 = String To Path(string=w888) -> (path=w886:path)
            n473 = Delete(path (use dialog)=w886) -> ()  [unwired: 4 in, 3 out]
          }
        }
      }
      frame "clear table 2" {
        n474 = property on="Cycle Name" class="Str (strict)"("Value"="" ("Subcycle name")) -> ()  [unwired: 2 in, 2 out]
        n475 = local write "Flag 2"(FALSE) -> ()
        n476 = local write "Cycle Pattern"(string[][] [["", "", "", "", ""], ["", "", "", "", ""], ["", "", "", "", ""], ["", "", "", "", ""], ["", "", "", "", ""], ["", "", "", "", ""], ["", "", "", "", ""], ["", "", "", "", ""], ["", "", "", "", ""], ["", "", "", "", ""], ["", "", "", "", ""], ["", "", "", "", ""], ["", "", "", "", ""], ["", "", "", "", ""], ["", "", "", "", ""], ["", "", "", "", ""], ["", "", "", "", ""], ["", "", "", "", ""], ["", "", "", "", ""], ["", "", "", "", ""], ["", "", "", "", ""], ["", "", "", "", ""], ["", "", "", "", ""], ["", "", "", "", ""], ["", "", "", "", ""], ["", "", "", "", ""], ["", "", "", "", ""], ["", "", "", "", ""], ["", "", "", "", ""], ["", "", "", "", ""], ["", "", "", "", ""]]) -> ()
      }
      frame "update list 2" {
        n477 = String To Path(string=w895) -> (path=w896:path)
        n478 = List Folder(path=w896, pattern="*.eyec") -> (filenames=w894:string[])  [unwired: 2 in, 3 out]
        n479 = property on="Cycle List" class="LstBox (strict)"("Item Names"=w894) -> ()  [unwired: 2 in, 2 out]
      }
      frame "save cycle" {
        w897 = ".eyec" ("string")
        n480 = local read "Cycle Name"() -> (w898:T5)
        n481 = String To Path(string=w910) -> (path=w911:path)
        n482 = List Folder(path=w911, pattern="*.eyec" ("string")) -> (filenames=w909:string[])  [unwired: 2 in, 3 out]
        n483 = Equal?(x=w898, y="") -> (x = y?=w904:bool)
        n484 = Concatenate Strings(w898, w897) -> (w900:string)
        n485 = Search 1D Array(1D array=w909, element=w900) -> (index of element=w908:i32)  [unwired: 1 in]
        n486 = Concatenate Strings(w910, w898, w897) -> (w913:string)
        n487 = case shown="True" w904 {
          tunnel: [TRUE FALSE] -> w902
          frame False {
          }
          frame True {
            n488 = One Button Dialog(message="Insert file name!") -> ()  [unwired: 1 in, 1 out]
          }
        }
        n489 = String To Path(string=w913) -> (path=w912:path)
        n490 = Equal?(x=w908, y=-1) -> (x = y?=w906:bool)
        n491 = case shown="False" w906 {
          selector: w906 -> [_ w962]
          tunnel: [w960 w962] -> w903
          frame False {
            n492 = Two Button Dialog(message="A file with this name already exists!\nDo you want to overwrite?") -> (T button?=w960:bool)  [unwired: 2 in]
          }
          frame True {
          }
        }
        n493 = And(x=w903, y=w902) -> (x .and. y?=w901:bool)
        n494 = case shown="True" w901 {
          tunnel: w912 -> [_ w920]
          frame False {
          }
          frame True {
            n495 = local read "Cycle Pattern"() -> (w919:string[][])
            n496 = call "Table check.vi"("Input table"=w919) -> ("Incomplete?"=w917:bool, "Length"=w918:i32)  [unwired: 9 in]
            n497 = case shown="False" w917 {
              tunnel: w920 -> [w929 _]
              tunnel: w919 -> [w928 _]
              tunnel: w918 -> [w921 _]
              frame False {
                n498 = Number To Decimal String(number=w921) -> (decimal integer string=w924:string)  [unwired: 1 in]
                n499 = for {
                  N: w921 -> [_]
                  tunnel: w928 -> [w958]
                  shift-right: [w946] -> w925
                  shift-left: string[] [] -> [w956]
                  i -> [w957]
                  w937 = 12 ("length")
                  n500 = Index Array(array=w958, index (row)=w957) -> (element=w952:string[])  [unwired: 1 in]
                  n501 = Index Array(array=w952, index=3) -> (element=w942:string)
                  n502 = Index Array(array=w952, index=1) -> (element=w941:string)
                  n503 = Concatenate Strings("C:\\Setup Files\\Subcycles Folder\\", w941) -> (w953:string)
                  n504 = String To Path(string=w953) -> (path=w954:path)
                  n505 = call-poly <vilib>:"Read From Spreadsheet File.vi"("file path (dialog if empty)"=w954) -> ("first row"=w945:string[])  [unwired: 6 in, 4 out]
                  n506 = Delete From Array(array=w945, length=1, index=0) -> (array with subset deleted=w939:string[])  [unwired: 1 out]
                  n507 = String Length(string=w939) -> (length=w948:i32[])
                  n508 = Array Size(array=w948) -> (size(s)=w940:i32)
                  n509 = Divide(x=w940, y=w937) -> (x/y=w938:dbl)
                  n510 = Decrement(x=w938) -> (x-1=w930:dbl)
                  n511 = Multiply(x=w937, y=w930) -> (x*y=w936:dbl)
                  n512 = Number To Decimal String(number=w930) -> (decimal integer string=w947:string)  [unwired: 1 in]
                  n513 = Delete From Array(array=w939, length=12, index=w936) -> (deleted portion=w933:string[], array with subset deleted=w934:string[])
                  n514 = Index Array(array=w933, index=0) -> (element=w931:string)
                  n515 = Build Array (concatenate)(w941, w942, w947, w931, w934) -> (w951:string[])
                  n516 = Build Array (concatenate)(w956, w951) -> (w946:string[])
                }
                n517 = local write "Flag 2"(FALSE) -> ()
                n518 = Build Array (concatenate)("Cycle Data File for EYECAT - do not modify", w924, w925) -> (w926:string[])
                n519 = call-poly <vilib>:"Write To Spreadsheet File.vi"("1D data"=w926, "file path (dialog if empty)"=w929) -> ()  [unwired: 6 in, 1 out]
              }
              frame True {
                n520 = One Button Dialog(message="The table is incomplete!\nplease review and save again!") -> ()  [unwired: 1 in, 1 out]
              }
            }
          }
        }
      }
      frame "load cycle" {
        n521 = local read "Flag 2"() -> (w966:bool)
        n522 = case shown="True" w966 {
          tunnel: [w1005 w1007] -> w963
          tunnel: w965 -> [w1005 w1007]
          tunnel: [TRUE ("T button?") w1006] -> w964
          frame False {
          }
          frame True {
            n523 = Two Button Dialog(message="The table has been modified.\nDo you want to continue?") -> (T button?=w1006:bool)  [unwired: 2 in]
          }
        }
        n524 = case shown="True" w964 {
          tunnel: w963 -> [_ w969]
          frame False {
          }
          frame True {
            n525 = property on="Cycle List" class="LstBox (strict)"() -> ("Item Names"=w985:string[])  [unwired: 2 in, 2 out]
            n526 = Index Array(array=w985, index="Cycle List") -> (element=w971:string)
            n527 = Concatenate Strings(w969, w971) -> (w984:string)
            n528 = Search/Split String(string=w971, search string/char (-)=".") -> (substring before match=w970:string)  [unwired: 1 in, 2 out]
            n529 = String To Path(string=w984) -> (path=w983:path)
            n530 = local write "Cycle Name"(w970) -> ()
            n531 = call-poly <vilib>:"Read From Spreadsheet File.vi"("file path (dialog if empty)"=w983) -> ("first row"=w967:string[])  [unwired: 6 in, 4 out]
            n532 = Delete From Array(array=w967, length=2, index=0) -> (array with subset deleted=w968:string[])  [unwired: 1 out]
            n533 = Index Array(array=w967, index=1) -> (element=w982:string)
            n534 = Decimal String To Number(string=w982) -> (number=w981:i32)  [unwired: 2 in, 1 out]
            n535 = for {
              N: w981 -> [_]
              tunnel: w968 -> [w1003]
              tunnel: [w998] -> w976 mode=indexing
              shift-right: [w988] -> _
              shift-left: 0 ("x") -> [w989]
              i -> [w1002]
              w999 = ""
              n536 = Increment(x=w989) -> (x+1=w987:i32)
              n537 = Increment(x=w987) -> (x+1=w995:i32)
              n538 = Increment(x=w1002) -> (x+1=w997:i32)
              n539 = Number To Decimal String(number=w997) -> (decimal integer string=w996:string)  [unwired: 1 in]
              n540 = Index Array(array=w1003, index #1=w989, index #2=w987, index #3=w995) -> (element #1=w1001:string, element #2=w1000:string, element #3=w994:string)
              n541 = Build Array(w996, w1001, w999, w1000, w999) -> (w998:string[])
              n542 = Decimal String To Number(string=w994) -> (number=w993:i32)  [unwired: 2 in, 1 out]
              n543 = Multiply(x=w993, y=12 ("x")) -> (x*y=w991:i32)
              n544 = Compound Arithmetic op=ADD(w991, 4, w989) -> (w988:i32)
            }
            n545 = Insert Into Array(array=string[][] [["", "", "", "", ""], ["", "", "", "", ""], ["", "", "", "", ""], ["", "", "", "", ""], ["", "", "", "", ""], ["", "", "", "", ""], ["", "", "", "", ""], ["", "", "", "", ""], ["", "", "", "", ""], ["", "", "", "", ""], ["", "", "", "", ""], ["", "", "", "", ""], ["", "", "", "", ""], ["", "", "", "", ""], ["", "", "", "", ""], ["", "", "", "", ""], ["", "", "", "", ""], ["", "", "", "", ""], ["", "", "", "", ""], ["", "", "", "", ""], ["", "", "", "", ""], ["", "", "", "", ""], ["", "", "", "", ""], ["", "", "", "", ""], ["", "", "", "", ""], ["", "", "", "", ""], ["", "", "", "", ""], ["", "", "", "", ""], ["", "", "", "", ""], ["", "", "", "", ""], ["", "", "", "", ""]], index (row)=0, new element=w976) -> (w975:string[][])  [unwired: 1 in]
            n546 = local write "Cycle Pattern"(w975) -> ()
          }
        }
      }
      frame "delete cycle" {
        n547 = Two Button Dialog(message="This operation will permanently delete this file!\nDo you want to continue?") -> (T button?=w1011:bool)  [unwired: 2 in]
        n548 = case shown="True" w1011 {
          tunnel: w1010 -> [_ w1016]
          frame False {
          }
          frame True {
            n549 = local read "Cycle List"() -> (w1017:i32)
            n550 = property on="Cycle List" class="LstBox (strict)"() -> ("Item Names"=w1018:string[])  [unwired: 2 in, 2 out]
            n551 = Index Array(array=w1018, index=w1017) -> (element=w1015:string)
            n552 = Concatenate Strings(w1016, w1015) -> (w1014:string)
            n553 = String To Path(string=w1014) -> (path=w1013:path)
            n554 = Delete(path (use dialog)=w1013) -> ()  [unwired: 4 in, 3 out]
            n555 = local write "Flag 2"(FALSE) -> ()
          }
        }
      }
      frame "calc HC CO" {
        n556 = local read "Sub-Cycle Pattern"() -> (w1035:string[][])
        n557 = Index Array(array=w1035, index (col) #1=3 ("disabled index (col)"), index (col) #2=4 ("index (col)"), index (col) #3=11 ("index (col)")) -> (element #1=w1025:string[], element #2=w1032:string[], element #3=w1019:string[])  [unwired: 3 in]
        n558 = Array Size(array=w1025) -> (size(s)=w1023:i32)
        n559 = Search 1D Array(1D array=w1025, element="") -> (index of element=w1022:i32)  [unwired: 1 in]
        n560 = Equal?(x=w1022, y=-1) -> (x = y?=w1024:bool)
        n561 = Select(t=w1023, s=w1024, f=w1022) -> (s? t:f=w1021:i32)
        n562 = for {
          N: w1021 -> [_]
          tunnel: [w1046] -> w1029 mode=indexing
          tunnel: [w1045] -> w1028 mode=indexing
          tunnel: w1025 -> [w1044] mode=indexing
          tunnel: w1032 -> [w1043] mode=indexing
          tunnel: w1019 -> [w1042] mode=indexing
          w1041 = ""
          n563 = Not Equal?(x=w1044, y=w1041) -> (x != y?=w1040:bool)
          n564 = Not Equal?(x=w1043, y=w1041) -> (x != y?=w1039:bool)
          n565 = Not Equal?(x=w1042, y=w1041) -> (x != y?=w1038:bool)
          n566 = Compound Arithmetic op=AND(w1040, w1039, w1038) -> (w1037:bool)
          n567 = case shown="True" w1037 {
            tunnel: w1044 -> [_ w1075]
            tunnel: w1043 -> [_ w1074]
            tunnel: [w1047 w1071] -> w1045
            tunnel: [w1047 w1070] -> w1046
            tunnel: w1042 -> [_ w1048]
            frame False {
              w1047 = ""
            }
            frame True {
              # "O2Eq"
              n568 = Fract/Exp String To Number(string=w1048) -> (number=w1049:dbl)  [unwired: 3 in, 1 out]
              n569 = Fract/Exp String To Number(string=w1075) -> (number=w1056:dbl)  [unwired: 3 in, 1 out]
              n570 = Fract/Exp String To Number(string=w1074) -> (number=w1052:dbl)  [unwired: 3 in, 1 out]
              n571 = Decrement(x=w1056) -> (x-1=w1057:dbl)
              n572 = Divide(x=w1049, y=20000.0) -> (x/y=w1050:dbl)
              n573 = Multiply(x=4.76, y=w1056) -> (x*y=w1061:dbl)
              n574 = Multiply(x=w1057, y=100.0) -> (x*y=w1059:dbl)
              n575 = Add(x=w1052, y=w1050) -> (x+y=w1053:dbl)
              n576 = Add(x=0.33, y=w1061) -> (x+y=w1063:dbl)
              n577 = Divide(x=w1059, y=w1063) -> (x/y=w1064:dbl)
              n578 = Subtract(x=w1053, y=w1064) -> (x-y=w1066:dbl)
              n579 = Multiply(x=w1066, y=2.0) -> (x*y=w1054:dbl)
              n580 = Divide(x=w1066, y=5.0) -> (x/y=w1055:dbl)
              n581 = Number To Fractional String(number=w1055, width (-)=i16 6, precision (6)=i16 3) -> (F-format string=w1070:string)  [unwired: 1 in]
              n582 = Number To Fractional String(number=w1054, width (-)=i16 6, precision (6)=i16 2) -> (F-format string=w1071:string)  [unwired: 1 in]
            }
          }
        }
        n583 = Replace Array Subset(array=w1035, new element #1=w1029, index (col) #1=5 ("disabled index (col)"), new element #2=w1028, index (col) #2=6 ("disabled index (col)")) -> (w1033:string[][])  [unwired: 2 in]
        n584 = local write "Sub-Cycle Pattern"(w1033) -> ()
      }
      frame "Total time calc" {
        w1090 = i16 2 ("width (-)")
        w1097 = ":"
        n585 = local read "Cycle Pattern"() -> (w1104:string[][])
        n586 = Index Array(array=w1104, index (col)=4 ("disabled index (col)")) -> (element=w1077:string[])  [unwired: 1 in]
        n587 = Array Size(array=w1077) -> (size(s)=w1079:i32)
        n588 = Search 1D Array(1D array=w1077, element="") -> (index of element=w1078:i32)  [unwired: 1 in]
        n589 = Equal?(x=w1078, y=-1) -> (x = y?=w1080:bool)
        n590 = Select(t=w1079, s=w1080, f=w1078) -> (s? t:f=w1076:i32)
        n591 = for {
          N: w1076 -> [_]
          tunnel: w1077 -> [w1112] mode=indexing
          shift-right: [w1114] -> w1100
          shift-left: 0 -> [w1115]
          n592 = xnode "Match Regular Expression"("input string"=w1112, "regular expression"=":" ("search string/char (-)")) -> ("before match"=w1111:string, "after match"=w1108:string)  [unwired: 4 in, 3 out]
          n593 = Decimal String To Number(string=w1111) -> (number=w1110:i32)  [unwired: 2 in, 1 out]
          n594 = Decimal String To Number(string=w1108) -> (number=w1107:i32)  [unwired: 2 in, 1 out]
          n595 = Multiply(x=w1110, y=60) -> (x*y=w1106:i32)
          n596 = Add(x=w1106, y=w1107) -> (x+y=w1105:i32)
          n597 = Add(x=w1105, y=w1115) -> (x+y=w1114:i32)
        }
        n598 = local read "Total Number of Cycles"() -> (w1101:T1)
        n599 = Multiply(x=w1100, y=w1101) -> (x*y=w1096:T1)
        n600 = Quotient & Remainder(x=w1096, y=3600.0) -> (x-y*floor(x/y)=w1083:T1, floor(x/y)=w1093:T1)
        n601 = Quotient & Remainder(x=w1083, y=60.0) -> (x-y*floor(x/y)=w1091:T1, floor(x/y)=w1092:T1)
        n602 = Number To Decimal String(number=w1093) -> (decimal integer string=w1098:string)  [unwired: 1 in]
        n603 = Number To Decimal String(number=w1092, width (-)=w1090) -> (decimal integer string=w1094:string)
        n604 = Number To Decimal String(number=w1091, width (-)=w1090) -> (decimal integer string=w1089:string)
        n605 = Concatenate Strings(w1098, w1097, w1094, w1097, w1089) -> (w1088:string)
        n606 = call <vilib>:"Search and Replace Pattern.vi"("string"=w1088, "regular expression (\"\")"=" " ("replace string (\"\")"), "replace string (\"\")"="0" ("replace string (\"\")"), "replace all? (F)"=TRUE) -> ("result string"=→"Total Test Duration (hrs)":string)  [unwired: 1 in, 1 out]
      }
      frame "update Cycle pattern " {
        n607 = local read "Cycle Pattern"() -> (w1243:string[][])
        n608 = Index Array(array=w1243, index (col)=1 ("disabled index (col)")) -> (element=w1228:string[])  [unwired: 1 in]
        n609 = String To Path(string=w1245) -> (path=w1246:path)
        n610 = Array Size(array=w1228) -> (size(s)=w1231:i32)
        n611 = Search 1D Array(1D array=w1228, element="") -> (index of element=w1230:i32)  [unwired: 1 in]
        n612 = List Folder(path=w1246, pattern="*.eyes") -> (filenames=w1244:string[])  [unwired: 2 in, 3 out]
        n613 = Equal?(x=w1230, y=-1) -> (x = y?=w1232:bool)
        n614 = Select(t=w1231, s=w1232, f=w1230) -> (s? t:f=w1229:i32)
        n615 = for {
          N: w1229 -> [_]
          tunnel: w1243 -> [w1262] mode=indexing
          tunnel: w1245 -> [w1255]
          tunnel: [w1257] -> w1238 mode=indexing
          tunnel: [w1259] -> w1242 mode=indexing
          tunnel: [w1256] -> w1239 mode=indexing
          tunnel: w1244 -> [w1254]
          tunnel: [w1249] -> w1235 mode=indexing
          n616 = Index Array(array=w1262, index #1=1 ("index"), index #2=3 ("index")) -> (element #1=w1253:string, element #2=w1258:string)
          n617 = Search 1D Array(1D array=w1254, element=w1253) -> (index of element=w1252:i32)  [unwired: 1 in]
          n618 = Not Equal?(x=w1252, y=-1) -> (x != y?=w1250:bool)
          n619 = case shown="True" w1250 {
            tunnel: [w1266 w1280] -> w1259
            tunnel: w1258 -> [_ w1276]
            tunnel: [w1266 w1274] -> w1257
            tunnel: [w1266 w1273] -> w1256
            tunnel: w1255 -> [_ w1272]
            tunnel: w1253 -> [w1265 w1271]
            tunnel: [w1264 w1271] -> w1249
            frame False {
              w1266 = "N/A" ("String")
              n620 = Concatenate Strings(w1265, " - File NOT AVAILABLE !!!" ("string")) -> (w1264:string)
            }
            frame True {
              w1284 = i16 2 ("width (-)")
              n621 = Concatenate Strings(w1272, w1271) -> (w1302:string)
              n622 = String To Path(string=w1302) -> (path=w1301:path)
              n623 = call <vilib>:"Search and Replace Pattern.vi"("string"=w1276, "regular expression (\"\")"="[a-x ]" ("format string"), "replace string (\"\")"="", "replace all? (F)"=TRUE) -> ("result string"=w1273:string)  [unwired: 1 in, 1 out]
              n624 = call-poly <vilib>:"Read From Spreadsheet File.vi"("file path (dialog if empty)"=w1301) -> ("first row"=w1270:string[])  [unwired: 6 in, 4 out]
              n625 = Delete From Array(array=w1270, length=1, index=0) -> (array with subset deleted=w1269:string[])  [unwired: 1 out]
              n626 = Array Size(array=w1269) -> (size(s)=w1300:i32)
              n627 = Equal?(x=w1273, y="") -> (x = y?=w1288:bool)
              n628 = Subtract(x=w1300, y=12) -> (x-y=w1298:i32)
              n629 = Select(t="0", s=w1288, f=w1273) -> (s? t:f=w1287:string)
              n630 = Index Array(array=w1269, index=w1298) -> (element=w1274:string)
              n631 = Decimal String To Number(string=w1287) -> (number=w1297:i32)  [unwired: 2 in, 1 out]
              n632 = Decimal String To Number(string=w1274) -> (number=w1296:i32)  [unwired: 2 in, 1 out]
              n633 = Multiply(x=w1297, y=w1296) -> (x*y=w1295:i32)
              n634 = Quotient & Remainder(x=w1295, y=60) -> (x-y*floor(x/y)=w1293:i32, floor(x/y)=w1292:i32)
              n635 = Number To Decimal String(number=w1293, width (-)=w1284) -> (decimal integer string=w1290:string)
              n636 = Number To Decimal String(number=w1292, width (-)=w1284) -> (decimal integer string=w1289:string)
              n637 = Concatenate Strings(w1289, ":", w1290) -> (w1283:string)
              n638 = call <vilib>:"Search and Replace Pattern.vi"("string"=w1283, "regular expression (\"\")"=" " ("replace string (\"\")"), "replace string (\"\")"="0" ("replace string (\"\")"), "replace all? (F)"=TRUE) -> ("result string"=w1280:string)  [unwired: 1 in, 1 out]
            }
          }
        }
        n639 = Replace Array Subset(array=w1243, new element #1=w1235, index (col) #1=1 ("disabled index (col)"), new element #2=w1238, index (col) #2=2 ("disabled index (col)"), new element #3=w1239, index (col) #3=3 ("disabled index (col)"), new element #4=w1242, index (col) #4=4 ("disabled index (col)")) -> (w1247:string[][])  [unwired: 4 in]
        n640 = local write "Cycle Pattern"(w1247) -> ()
      }
      frame "load cycle name" {
        n641 = property on="Cycle Pattern" class="Tbl (strict)"() -> ("EditPos"=w1308:T3)  [unwired: 2 in, 2 out]
        n642 = Unbundle By Name(w1308) -> ("Row"=w1306:i32, "Column"=w1305:i32)
        n643 = local read "Cycle Pattern"() -> (w1304:string[][])
        n644 = call "SubCycles list.vi"() -> ("Subcycle name"=w1307:string)  [unwired: 10 in, 1 out]
        n645 = Replace Array Subset(array=w1304, new element=w1307, index (row)=w1306, index (col)=w1305) -> (w1303:string[][])
        n646 = local write "Cycle Pattern"(w1303) -> ()
      }
      frame "load test array" {
        n647 = local read "Total Test Duration (hrs)"() -> (w1316:T8)
        n648 = local read "Cycle Name"() -> (w1312:T5)
        n649 = Equal?(x=w1312, y="") -> (x = y?=w1311:bool)
        n650 = Not Equal?(x=w1316, y="0:00:00") -> (x != y?=w1310:bool)
        n651 = Or(x=w1310, y=w1311) -> (x .or. y?=w1309:bool)
        n652 = case shown="True" w1309 {
          selector: w1309 -> [w1317 _]
          tunnel: [FALSE TRUE] -> w1314
          frame False {
            n653 = case shown="False" w1317 {
              frame False {
                n654 = One Button Dialog(message="Incomplete Data!\nReview the cycle pattern!") -> ()  [unwired: 1 in, 1 out]
              }
              frame True {
              }
            }
          }
          frame True {
            w1323 = 0.0 ("default (0 I32)")
            n655 = local read "Cycle Name"() -> (w1338:T5)
            n656 = Concatenate Strings("C:\\Setup Files\\Cycles Folder\\", w1338, ".eyec" ("string")) -> (w1336:string)
            n657 = String To Path(string=w1336) -> (path=w1337:path)
            n658 = local read "Total Number of Cycles"() -> (w1334:T1)
            n659 = call-poly <vilib>:"Read From Spreadsheet File.vi"("file path (dialog if empty)"=w1337) -> ("first row"=w1320:string[])  [unwired: 6 in, 4 out]
            n660 = call "Remove names.vi"("Array in"=w1320) -> ("Array out"=w1329:string[])  [unwired: 10 in]
            n661 = Index Array(array=w1320, index #1=14 ("index"), index #2=15 ("index")) -> (element #1=w1325:string, element #2=w1321:string)
            n662 = Number To Decimal String(number="Ageing Gas") -> (decimal integer string=w1333:string)  [unwired: 1 in]
            n663 = Number To Decimal String(number=w1334) -> (decimal integer string=w1332:string)  [unwired: 1 in]
            n664 = Decimal String To Number(string=w1321, default (0L)=w1323) -> (number=w1322:dbl)  [unwired: 1 in, 1 out]
            n665 = Decimal String To Number(string=w1325, default (0L)=w1323) -> (number=w1324:dbl)  [unwired: 1 in, 1 out]
            n666 = property on="Inlet temp Age" class="DigNum (strict)"("Value"=w1324) -> ()  [unwired: 2 in, 2 out]
            n667 = property on="Flow rate Age" class="DigNum (strict)"("Value"=w1322) -> ()  [unwired: 2 in, 2 out]
            n668 = Build Array (concatenate)(w1333, w1332, w1329) -> (w1328:string[])
            n669 = shared-variable "My Computer\\Library 1.lvlib\\Ageing Variables"(w1328) -> ()  [unwired: 1 in, 1 out]
          }
        }
        "Test Compiled" <- w1314
      }
      frame "convert to num" {
        n670 = local read "EditPos Subc"() -> (w1343:T3)
        n671 = Unbundle By Name(w1343) -> ("Row"=w1344:i32, "Column"=w1341:i32)
        n672 = Equal?(x=w1341, y=7) -> (x = y?=w1340:bool)
        n673 = case shown="False" w1340 {
          tunnel: w1344 -> [_ w1349]
          tunnel: w1341 -> [_ w1347]
          tunnel: w1343 -> [_ _]
          frame True {
          }
          frame False {
            n674 = local read "Sub-Cycle Pattern"() -> (w1346:string[][])
            n675 = call "Conv to num.vi"("Column"=w1347, "Row"=w1349, "Array"=w1346) -> ("result string"=w1348:string)  [unwired: 8 in]
            n676 = Replace Array Subset(array=w1346, new element=w1348, index (row)=w1349, index (col)=w1347) -> (w1345:string[][])
            n677 = local write "Sub-Cycle Pattern"(w1345) -> ()
          }
        }
      }
      frame "check scycle name" {
        n678 = local read "Sub-Cycle Name"() -> (w1350:T5)
        n679 = call <vilib>:"Search and Replace Pattern.vi"("string"=w1350, "regular expression (\"\")"="[^0-9a-zA-Z ]" ("format string"), "replace string (\"\")"="", "replace all? (F)"=TRUE) -> ("result string"=w1356:string)  [unwired: 1 in, 1 out]
        n680 = Not Equal?(x=w1356, y=w1350) -> (x != y?=w1355:bool)
        n681 = case shown="False" w1355 {
          tunnel: w1356 -> [w1357 w1358]
          tunnel: [w1357 w1358] -> w1351
          frame False {
          }
          frame True {
            n682 = One Button Dialog(message="Unsuitable character for the file name!") -> ()  [unwired: 1 in, 1 out]
          }
        }
        n683 = local write "Sub-Cycle Name"(w1351) -> ()
      }
      frame "check cycle name" {
        n684 = local read "Cycle Name"() -> (w1360:T5)
        n685 = call <vilib>:"Search and Replace Pattern.vi"("string"=w1360, "regular expression (\"\")"="[^0-9a-zA-Z ]" ("format string"), "replace string (\"\")"="", "replace all? (F)"=TRUE) -> ("result string"=w1366:string)  [unwired: 1 in, 1 out]
        n686 = Not Equal?(x=w1366, y=w1360) -> (x != y?=w1365:bool)
        n687 = case shown="False" w1365 {
          tunnel: w1366 -> [w1367 w1368]
          tunnel: [w1367 w1368] -> w1361
          frame False {
          }
          frame True {
            n688 = One Button Dialog(message="Unsuitable character for the file name!") -> ()  [unwired: 1 in, 1 out]
          }
        }
        n689 = local write "Cycle Name"(w1361) -> ()
      }
      frame "Multigas connect" {
        # "add here logic to verify the user requirements and the machine state\n0 - not connected\n1 - MKS1 & Ext An Up\n2 - MKS2 & Ext An Dn\n3 - MKS 1 & 2  & Ext An Up & Dn"
        n690 = flat-sequence {
          frame #0 {
            "Connected?" <- TRUE
          }
        }
      }
      frame "Multigas disconnect" {
      }
    }
    n691 = local read "stop 2"() -> (w746:bool)
  }
  n692 = node-c288(w1) -> ()  [unwired: 1 out]
  n693 = local write "stop 2"(w11) -> ()
  n694 = disable-structure shown="Disabled" {
    frame Disabled {
      n695 = while {
        tunnel: [w1409] -> w1394
        tunnel: [w1408] -> w1393
        stop <- w1405 stop-if-true
        n696 = TCP Open Connection(address="192.168.1.3", remote port or service name=u16 7700) -> (connection ID=w1409:refnum<k5>, error out=w1408:errorcluster)  [unwired: 3 in]
        n697 = Unbundle By Name(w1408) -> ("status"=w1410:bool)
        n698 = Not(x=w1410) -> (.not. x?=w1406:bool)
        n699 = Or(x=w1406, y="stop TCP") -> (x .or. y?=w1405:bool)
      }
      n700 = Concatenate Strings("\r", "\n") -> (w1382:string)
      n701 = Concatenate Strings("MSSM,0,1,1" ("data in"), w1382) -> (w1389:string)
      n702 = TCP Write(connection ID=w1394, data in=w1389, error in (no error)=w1393) -> (connection ID out=w1397:refnum<k5>, error out=w1398:errorcluster)  [unwired: 1 in, 1 out]
      n703 = Concatenate Strings("MSMD,1,7,1,1,1,1,2,1,1,3,1,1,4,1,1,5,1,1,6,1,1,7,1" ("data in"), w1382) -> (w1384:string)
      n704 = TCP Write(connection ID=w1397, data in=w1384, error in (no error)=w1398) -> (connection ID out=w1395:refnum<k5>, error out=w1396:errorcluster)  [unwired: 1 in, 1 out]
      n705 = Concatenate Strings("MSTT,1,0" ("string"), w1382) -> (w1383:string)
      n706 = TCP Write(connection ID=w1395, data in=w1383, error in (no error)=w1396) -> (connection ID out=w1381:refnum<k5>, error out=w1380:errorcluster)  [unwired: 1 in, 1 out]
      n707 = UDP Open(9:500 ("timeout ms (25000)"), 11:u16 7701 ("port")) -> ()  [unwired: 3 in, 3 out]
      n708 = UDP Read(timeout ms (25000)=500) -> (data out=w1372:string)  [unwired: 3 in, 4 out]
      n709 = while {
        shift-right: [w1401] -> _
        shift-left: w1372 -> [w1404]
        tunnel: [w1402] -> w1373 mode=indexing
        stop <- w1399 stop-if-true
        n710 = Search/Split String(string=w1404, search string/char (-)=",") -> (substring before match=w1402:string, match + rest of string=w1401:string)  [unwired: 1 in, 1 out]
        n711 = String Length(string=w1401) -> (length=w1400:i32)
        n712 = Equal To 0?(x=w1400) -> (x = 0?=w1399:bool)
      }
      n713 = call "7170string to array.vi"("Array in"=w1373) -> ()  [unwired: 4 in, 1 out]
      n714 = UDP Close() -> ()  [unwired: 2 in, 2 out]
      n715 = Concatenate Strings("MSTP,0,0" ("string"), "\r", "\n") -> (w1376:string)
      n716 = TCP Write(data in=w1376) -> (connection ID out=w1378:refnum<k5>, error out=w1379:errorcluster)  [unwired: 3 in, 1 out]
      n717 = TCP Close Connection(connection ID=w1378, error in (no error)=w1379) -> ()  [unwired: 1 in, 2 out]
    }
    frame Enabled {
    }
  }
  n718 = node-c288(w8) -> ()  [unwired: 1 out]
  "Table" <- string[][] [] ("Table")
